vi "Text control 2 v6.8.vi"() -> ()   [LabVIEW 2016]
panel:
  in  "Tab Control":enum32{"Main", "Other parameters"}(tab)
  in  "Plot sample extrema vs time":bool
  out "Line running":i32
  out "Total lines":i32
  out "Path":path=path "C:/users/rlp38/09Apr2009LTtesting/test2.txt"
  out "I vs Vg":cluster{"Y data in":dbl[], "X data in":dbl[]}[](graph)
  out "Is max":dbl format="%.2e"
  out "Id max":dbl format="%.2e"
  out "Ig max":dbl format="%.2e"
  out "Imax vs time":cluster{"Y data in":dbl[], "X data in":dbl[]}[](graph)
  out "Imin vs time":cluster{"Y data in":dbl[], "X data in":dbl[]}[](graph)
  out "I vs Vd":cluster{"Y data in":dbl[], "X data in":dbl[]}[](graph)
  in  "Script":string="#pulsedstressV d 0.03 20 0 0.5 0.0827 5\n#\n#itime m\n#gaterangemode a\n#drainrangemode a\n#pulsed on 0.05 0 0.02\n#transfer d -10 40 1 5 40 35\n#transfer d -10 40 1 5 40 35\n#transfer d -10 40 1 5 40 35\n#output d 0 40 20 0 40 1\n#\n#\n#sample 1 0.008 221 6 0.003\n#samplei 400e-6 200 6 0.002 0.1\n#vsu2pulse -10 4\n#\n#stressV 0.016 0.03 2e-4 0.1e-3 11\n#stressI 220e-7 0.08 15\n#transfer s -1 1 0.5 -0.005 0.005 0.005\n#output s 0 0 0 -0.008 0.008 0.002"
  out "Command running:":string
  out "Serial port data":string
  out "Elapsed Time":dbl caption="Elapsed Time (s)"
  in  "Time Units":u16(ring)=1 items=["Seconds", "Minutes", "Hours"]
  in  "Time Offset":dbl caption="Set Start Time (s)"
  in  "Reset":bool
  in  "Auto Reset":bool
  in  "integration time":u32(slide) max=2 step=1 scale=0.0..2.0
  out "Is on":dbl format="%.2e"
  out "Id on":dbl format="%.2e"
  out "Ig on":dbl format="%.2e"
  out "Ion vs time":cluster{"Y data in":dbl[], "X data in":dbl[]}[](graph)
  out "Ioff vs time":cluster{"Y data in":dbl[], "X data in":dbl[]}[](graph)
  out "Ig min":dbl format="%.2e"
  out "Id min":dbl format="%.2e"
  out "Is min":dbl format="%.2e"
  out "Is off":dbl format="%.2e"
  out "Id off":dbl format="%.2e"
  out "Ig off":dbl format="%.2e"
  in  "Integration time (long)":dbl=0.32 min=0.04 max=2.0 step=0.02 format="%.2f"
  in  "Integration time (short)":dbl=0.0019 min=8e-05 max=0.0019 step=8e-05 format="%^.0e"
  in  "Drain: Compliance":dbl=0.001 format="%.8f"
  in  "Gate: Compliance":dbl=0.001 format="%.8f"
  in  "Interrupt scan":bool
  in  "Interrupt program":bool
  in  "Plot output curve extrema vs time":bool
  in  "Plot transfer curve extrema vs time":bool
  out "I vs time (Bias Stress)":cluster{"Y data in":dbl[], "X data in":dbl[]}[](graph)
  in  "Sample I - Probe 4 (Disabled)":u32(ring)=3 items=["SMU1  ", "SMU2  ", "SMU3  ", "SMU4  ", "SMU5  ", "SMU6  "]
  in  "Sample I - Source/Common":u32(ring) items=["SMU1  ", "SMU2  ", "SMU3  ", "SMU4  ", "SMU5  ", "SMU6  "]
  in  "Sample I - Probe 3 (Disabled)":u32(ring)=2 items=["SMU1  ", "SMU2  ", "SMU3  ", "SMU4  ", "SMU5  ", "SMU6  "]
  in  "Sample I - Drain/Gate":u32(ring)=1 items=["SMU1  ", "SMU2  ", "SMU3  ", "SMU4  ", "SMU5  ", "SMU6  "]
  in  "Sample - Probe 4":u32(ring)=3 items=["SMU1  ", "SMU2  ", "SMU3  ", "SMU4  ", "SMU5  ", "SMU6  "]
  in  "Sample - Source/Common":u32(ring) items=["SMU1  ", "SMU2  ", "SMU3  ", "SMU4  ", "SMU5  ", "SMU6  "]
  in  "Sample - Gate":u32(ring)=2 items=["SMU1  ", "SMU2  ", "SMU3  ", "SMU4  ", "SMU5  ", "SMU6  "]
  in  "Sample - Drain":u32(ring)=1 items=["SMU1  ", "SMU2  ", "SMU3  ", "SMU4  ", "SMU5  ", "SMU6  "]
  in  "Gate Range\nmode":u16(ring) items=["Auto", "Limited", "Fixed"]
  in  "Gate Range":u8(slide)=3 max=11 scale=0.0..11.0
  in  "Source/Drain\nRange mode":u16(ring) items=["Auto", "Limited", "Fixed"]
  in  "Source/Drain Range":u8(slide)=3 max=11 scale=0.0..11.0
  in  "Panel Controls":T1={"Emergency Stop"=refnum, "TransGraph Max"=1e-05, "Text/Graph (text=false)"=TRUE} {"TransGraph Max" format="%.2e"}
  in  "Panel Controls 2":T2={"Emergency Stop"=refnum, "TransGraph Max"=1e-05, "Text/Graph (text=false)"=TRUE, "TransGraph Min"=1e-11} {"TransGraph Min" format="%.2e"; "TransGraph Max" format="%.2e"}
  out "error out":errorcluster
  in  "Delay before read (ms)":u32=1000
  in  "byte count":u32=64
  in  "Serial End Mode for Reads":u16(ring)=2 items=["None", "LastBit", "TermChar"]
  in  "Timeout (ms)":u32=10000
  in  "Enable Termination\nChar (T)":bool=TRUE
  in  "Termination char\n(0xA = '\\n' = LF)\n(0xD = '\\r' = CR)":u8=13 format="%.0x"
  in  "flow control":u16(ring) items=["None"=0, "XON/XOFF"=1, "RTS/CTS"=2, "DTR/DSR"=4]
  in  "stop bits":u16(ring)=10 items=["1.0"=10, "1.5"=15, "2.0"=20]
  in  "parity":u16(ring) items=["None", "Odd", "Even", "Mark", "Space"]
  in  "data bits":u16=8 min=5 max=8 step=1
  in  "VISA resource name":refnum<visa-resource-name>="COM6"
  in  "baud rate":u32=9600
  out "Timings Indicator":T3
  in  "Timings (overwritten by the Front Panel)":T4={"integration time"=0, "Short/Long integration time"=0.00064, "hold time (sec)"=0.0, "delay time (sec)"=0.0, "Step Time (0 disables)"=0.0, "sweep method"=0, "Pulse period"=0.005, "Base voltage"=0.0, "Pulse width"=0.0005} {"Pulse width" min=0.0005 max=0.1 step=0.0001 format="%.4f"; "Base voltage" format="%^.4e"; "Pulse period" min=0.005 max=1.0 step=0.0001 format="%.4f"; "sweep method" items=["Continuous", "Pulsed"]; "Step Time (0 disables)" format="%.2f"; "delay time (sec)" format="%.4f"; "hold time (sec)" format="%.4f"; "Short/Long integration time" format="%^.0e"; "integration time" scale=0.0..2.0}
  in  "Probe 4":cluster{"on/off":bool, "Voltage":dbl} {"Voltage" min=-100.0 max=100.0 format="%.2f"}
  in  "Full Reset":bool
  in  "Standby":T5
  out "Probe 4 Indicator":cluster{"on/off":bool, "Voltage":dbl} {"Voltage" min=-100.0 max=100.0 format="%.2f"}
  in  "Transfer/Output - Drain":u32(ring)=1 items=["SMU1  ", "SMU2  ", "SMU3  ", "SMU4  ", "SMU5  ", "SMU6  "]
  in  "Transfer/Output - Gate":u32(ring)=2 items=["SMU1  ", "SMU2  ", "SMU3  ", "SMU4  ", "SMU5  ", "SMU6  "]
  in  "Transfer/Output - Source/Common":u32(ring) items=["SMU1  ", "SMU2  ", "SMU3  ", "SMU4  ", "SMU5  ", "SMU6  "]
  in  "Transfer/Output - Probe 4":u32(ring)=3 items=["SMU1  ", "SMU2  ", "SMU3  ", "SMU4  ", "SMU5  ", "SMU6  "]
  in  "Pulsed Stress V - Probe 4":u32(ring)=3 items=["SMU1  ", "SMU2  ", "SMU3  ", "SMU4  ", "SMU5  ", "SMU6  "]
  in  "Pulsed Stress V - Vextra":u32(ring)=1 items=["VSU1  ", "VSU2  "]
  in  "Pulsed Stress V - Drain":u32(ring)=1 items=["SMU1  ", "SMU2  ", "SMU3  ", "SMU4  ", "SMU5  ", "SMU6  "]
  in  "Pulsed Stress V - Source/Common":u32(ring) items=["SMU1  ", "SMU2  ", "SMU3  ", "SMU4  ", "SMU5  ", "SMU6  "]
  in  "Pulsed Stress V - Gate":u32(ring)=2 items=["SMU1  ", "SMU2  ", "SMU3  ", "SMU4  ", "SMU5  ", "SMU6  "]
  in  "FPP - Drain":u32(ring)=1 items=["SMU1  ", "SMU2  ", "SMU3  ", "SMU4  ", "SMU5  ", "SMU6  "]
  in  "FPP - Gate":u32(ring)=2 items=["SMU1  ", "SMU2  ", "SMU3  ", "SMU4  ", "SMU5  ", "SMU6  "]
  in  "FPP - Probe 1":u32(ring) items=["SMU1  ", "SMU2  ", "SMU3  ", "SMU4  ", "SMU5  ", "SMU6  "]
  in  "FPP - Probe 2":u32(ring)=3 items=["SMU1  ", "SMU2  ", "SMU3  ", "SMU4  ", "SMU5  ", "SMU6  "]
  in  "FPP - Source":u32(ring) items=["VSU1  ", "VSU2  "]
  in  "Stress V - Drain":u32(ring)=1 items=["SMU1  ", "SMU2  ", "SMU3  ", "SMU4  ", "SMU5  ", "SMU6  "]
  in  "Stress V - Gate":u32(ring)=2 items=["SMU1  ", "SMU2  ", "SMU3  ", "SMU4  ", "SMU5  ", "SMU6  "]
  in  "Stress V - Source/Common":u32(ring) items=["SMU1  ", "SMU2  ", "SMU3  ", "SMU4  ", "SMU5  ", "SMU6  "]
  in  "Stress I - Drain/Gate":u32(ring)=1 items=["SMU1  ", "SMU2  ", "SMU3  ", "SMU4  ", "SMU5  ", "SMU6  "]
  in  "Stress I - Source/Common":u32(ring) items=["SMU1  ", "SMU2  ", "SMU3  ", "SMU4  ", "SMU5  ", "SMU6  "]
  in  "VSU2 Stress - Source/Common":u32(ring) items=["SMU1  ", "SMU2  ", "SMU3  ", "SMU4  ", "SMU5  ", "SMU6  "]
  in  "VISA resource name in":refnum<visa-resource-name>="GPIB0::14::INSTR"
  in  "Gate":T6={"Gate Start"=0.0, "Gate Stop"=2.0, "Gate Step (linear only)"=1.0, "Gate Compliance"=0.0001, "Gate PComp"=0.0, "Range mode"=0, "Range"=6} {"Range" max=11 scale=0.0..11.0; "Range mode" items=["Auto", "Limited", "Fixed"]; "Gate PComp" format="%^.2e"; "Gate Compliance" format="%^.2e"; "Gate Step (linear only)" format="%^.4e"; "Gate Stop" format="%^.4e"; "Gate Start" format="%^.4e"}
  in  "Drain 2":T7={"Drain Start"=0.0, "Drain Stop"=2.0, "Drain Compliance"=0.0001, "Drain Step"=1.0, "Drain PComp"=0.0, "Range mode"=0, "Range"=6} {"Range" max=11 scale=0.0..11.0; "Range mode" items=["Auto", "Limited", "Fixed"]; "Drain PComp" format="%^.2e"; "Drain Step" format="%^.4e"; "Drain Compliance" format="%^.2e"; "Drain Stop" format="%^.4e"; "Drain Start" format="%^.4e"}
  # "Time"
  # "Syntax:\nitime [s|m|l] time(sec): [s|m|l] determines the integration time setting (small|medium|long) and time sets the value.\nNOTE: The value of the integration time has to be within the range allowed by its category (s|m|l), otherwise, the closest value will be used. (e.g. if the category is set to short but the time value is very long, the actual value used will be the maximum short integration time.\nIntegration times:\n    Short: Default: 640 us. Range: 8E-5 - 1.92E-3 seconds.\n    Medium: Fixed at 1 NPL cycle (0.02 seconds).\n    Long: Default: 16 NPL cycles (0.32 seconds). Range: 2-100 NPL cycles (0.04 seconds - 2 seconds).\ngaterangemode [a|l|f]\ndrainrangemode [a|l|f]\npulsed [on|off] PulsePeriod(sec) PulseBaseVoltage PulseONWidth(sec)\nstandby [on l off]\nwait NumMilliseconds\nwait-min NumMinutes\n# texthere = comment\nProbe4 [ON|OFF] Voltage\ntransfer [s|d] VgStart VgStop VgStep VdStart VdStop VdStep\noutput [s|d] VgStart VgStop VgStep VdStart VdStop VdStep\nsample Vg Vd NumSamples Time(s) SampleInterval(s)\nsamplei Idg NumSamples Time(s) SampleInterval(s) VDGcompliance\n100 samples is approximately 13 seconds with medium integration\n# if in doubt use SampleInterval(s) = 0.004\n    NOTE: When doing bias stress measurements, set the Time Units to \"Seconds\", as the \"sample\" command has been configured to give the output to seconds.\nstressV VG VD IGcompliance IDcompliance Duration(sec)\nstressI IDG VDGcompliance Duration(sec)\nvsu2pulse Bias Duration(s)\npulsedstressV [s|d] VEstop VgON VgOFF Period(s) PulseONwidth(s) Vd\nsample-fpp Vg Vd NumSamples Time\nresample-fpp Vg Vd\ntransfer-fpp [s|d] VgStart VgStop VgStep VdStart VdStop VdStep\noutput-fpp [s|d] VgStart VgStop VgStep VdStart VdStop VdStep\nserial SerialPortCommand"
  # "1\n2\n3\n4\n5\n6\n7\n8\n9\n10\n11\n12\n13\n14\n15\n16\n17\n18\n19\n20"
  # "SMUs"
  # "Serial port settings"
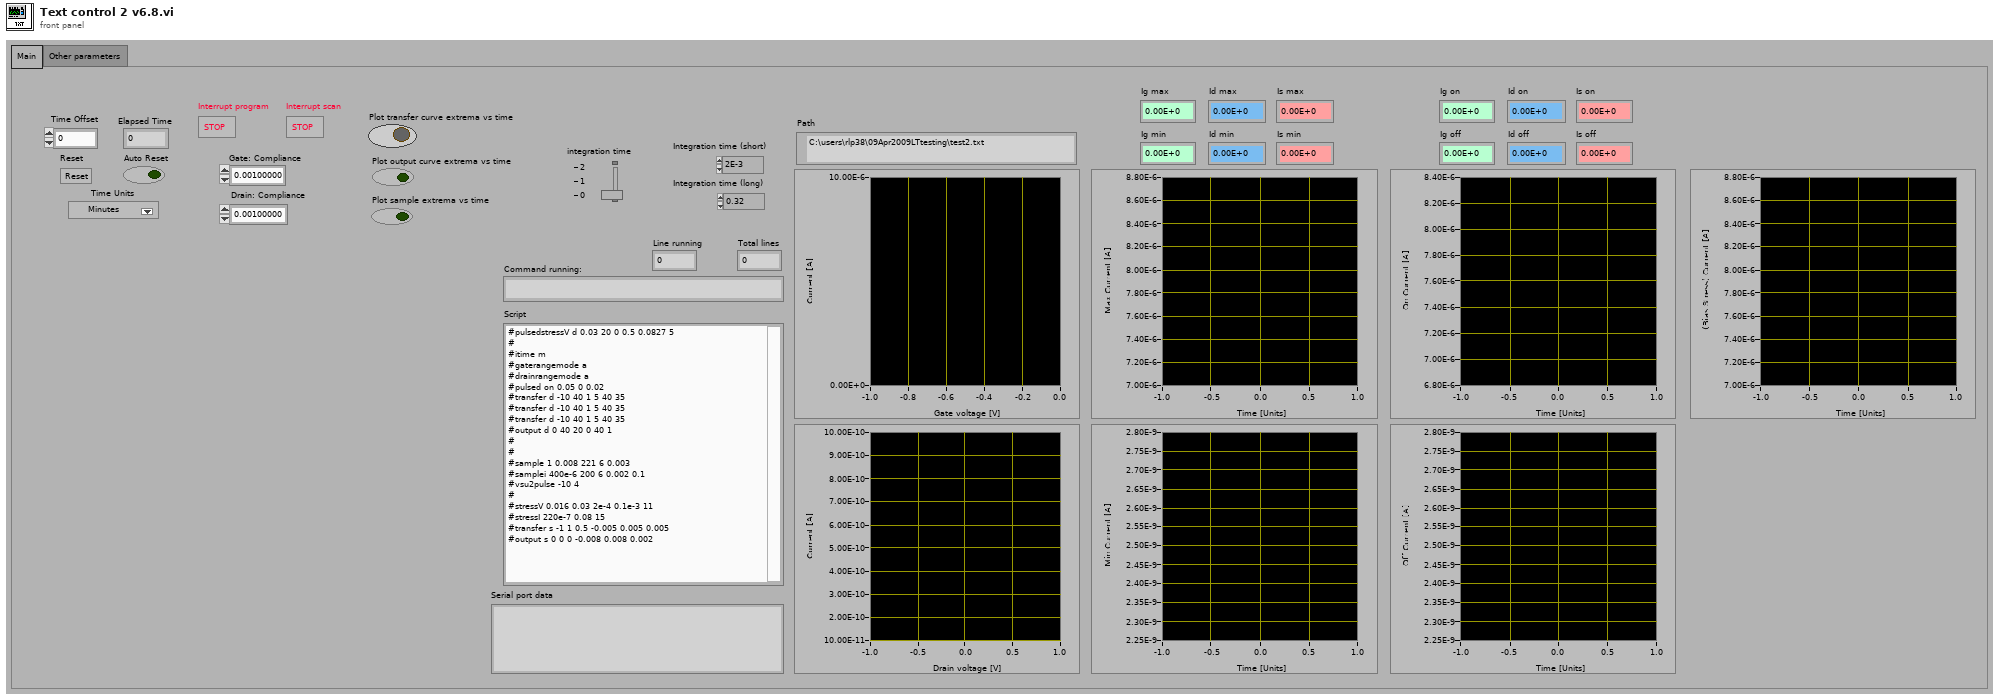
[diagram p1: front panel]
types:
  T1 = cluster{"Emergency Stop":refnum<vi>, "TransGraph Max":dbl, "Text/Graph (text=false)":bool}
  T2 = cluster{"Emergency Stop":refnum<vi>, "TransGraph Max":dbl, "Text/Graph (text=false)":bool, "TransGraph Min":dbl}
  T3 = cluster{"integration time (0:s, 1:m, 2:l)":u32, "Short/Long integration time":dbl, "hold time (sec)":dbl, "delay time (sec)":dbl, "Step Time (0 disables)":dbl, "sweep method":u16, "Pulse period":dbl, "Base voltage":dbl, "Pulse width":dbl}
  T4 = cluster{"integration time":u32, "Short/Long integration time":dbl, "hold time (sec)":dbl, "delay time (sec)":dbl, "Step Time (0 disables)":dbl, "sweep method":u16, "Pulse period":dbl, "Base voltage":dbl, "Pulse width":dbl}
  T5 = cluster{"Gate Standby":bool, "Drain Standby":bool}
  T6 = cluster{"Gate Start":dbl, "Gate Stop":dbl, "Gate Step (linear only)":dbl, "Gate Compliance":dbl, "Gate PComp":dbl, "Range mode":u16, "Range":u8}
  T7 = cluster{"Drain Start":dbl, "Drain Stop":dbl, "Drain Compliance":dbl, "Drain Step":dbl, "Drain PComp":dbl, "Range mode":u16, "Range":u8}
  T8 = enum16{"open", "replace", "create", "open or create", "replace or create", "replace or create with confirmation"}
  T9 = cluster{"V2 Start":dbl, "V2 Step":dbl, "Number of points":i32}
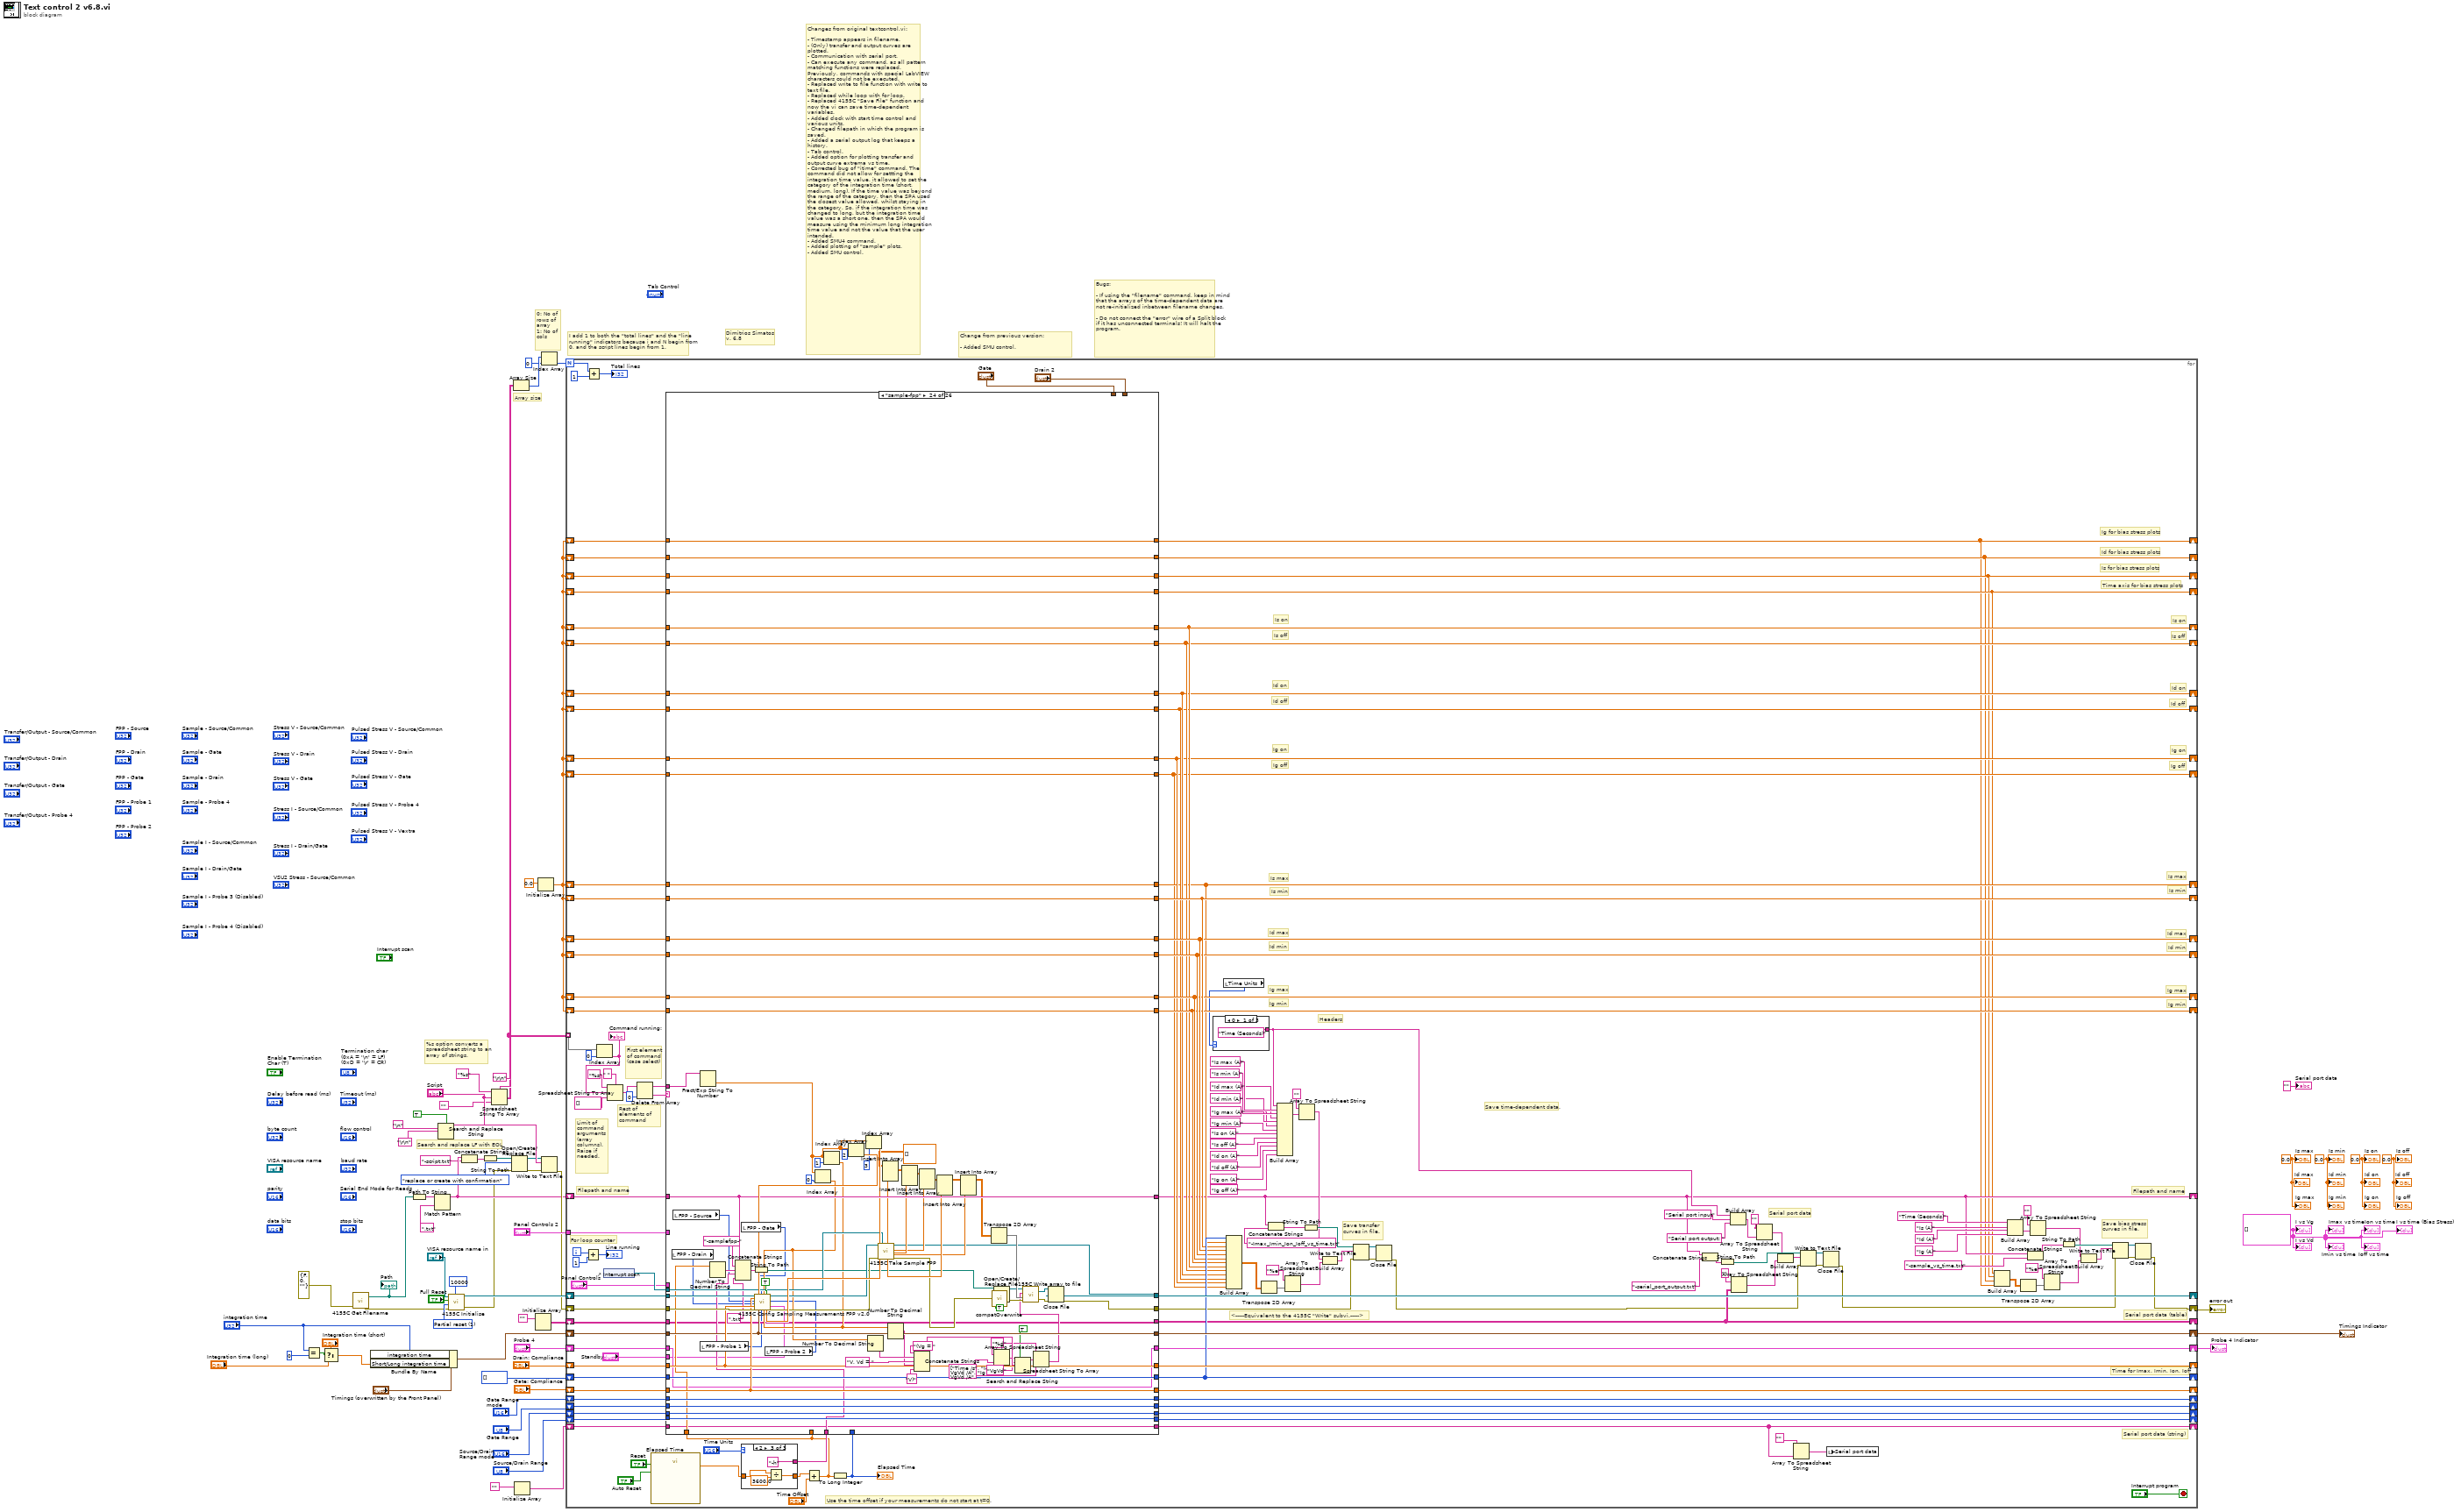
[diagram p0: block diagram]
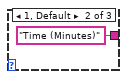
[diagram p2: hidden frame]
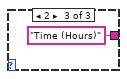
[diagram p3: hidden frame]
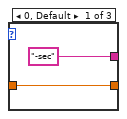
[diagram p4: hidden frame]
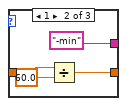
[diagram p5: hidden frame]
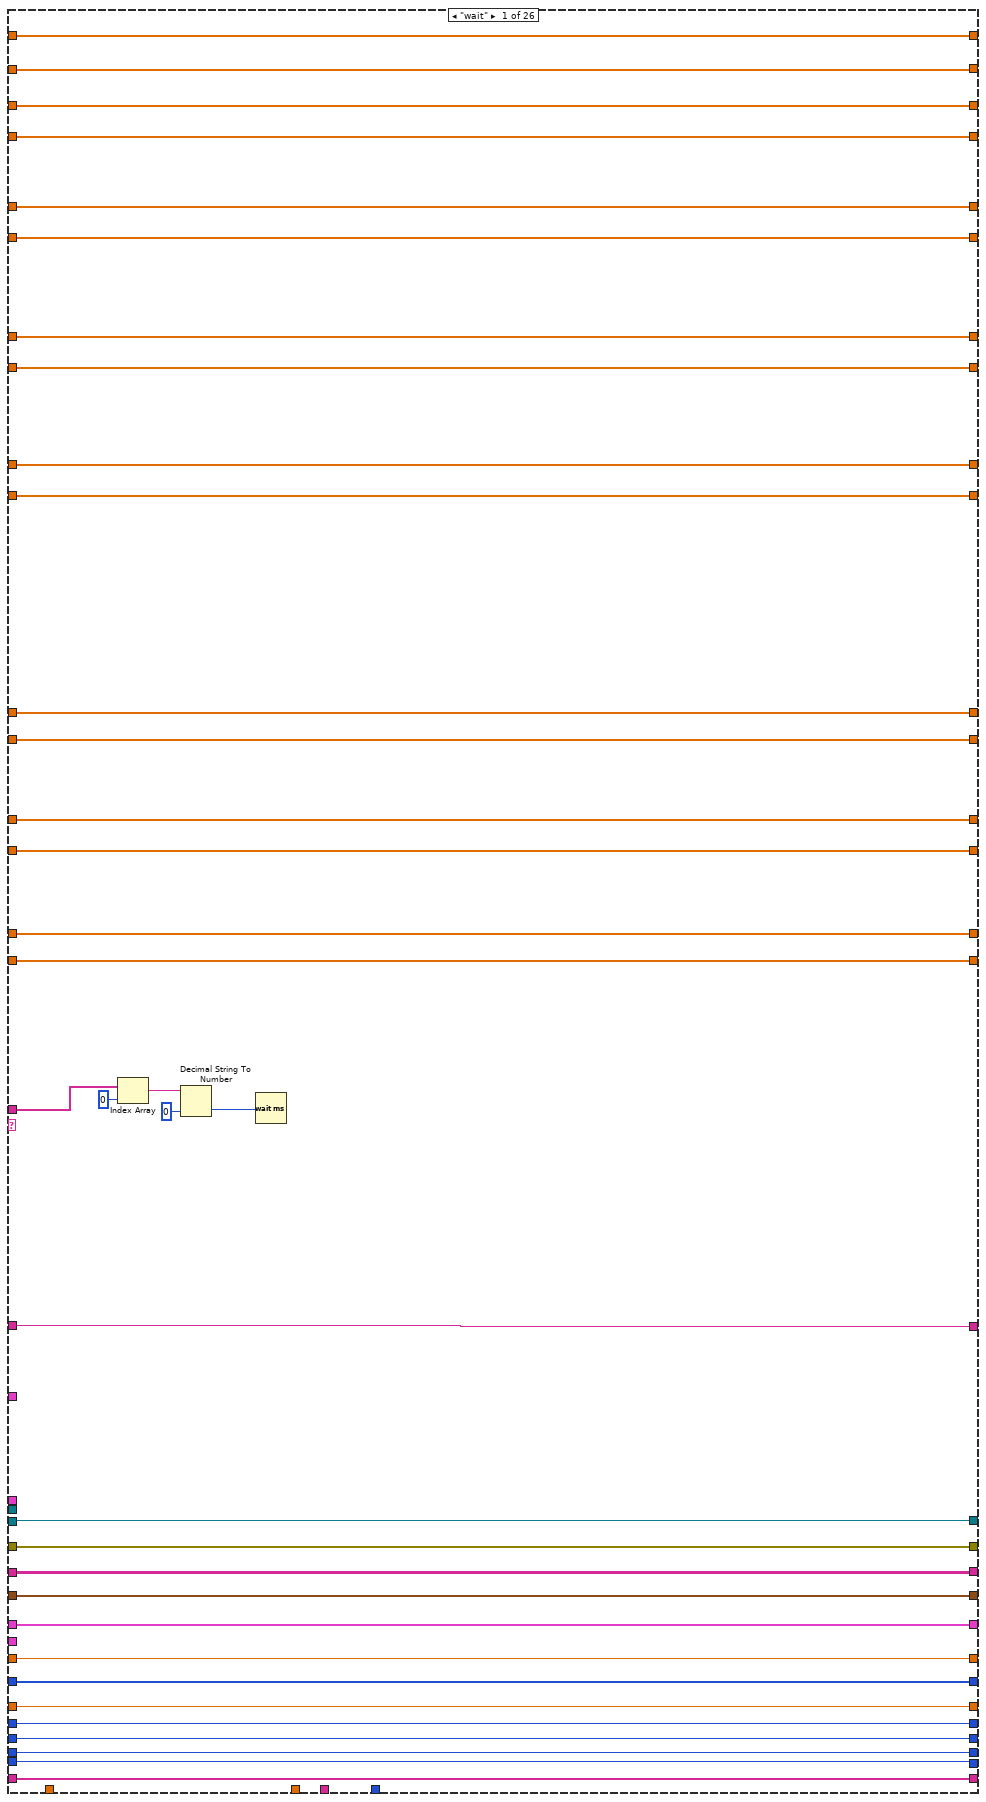
[diagram p6: hidden frame]
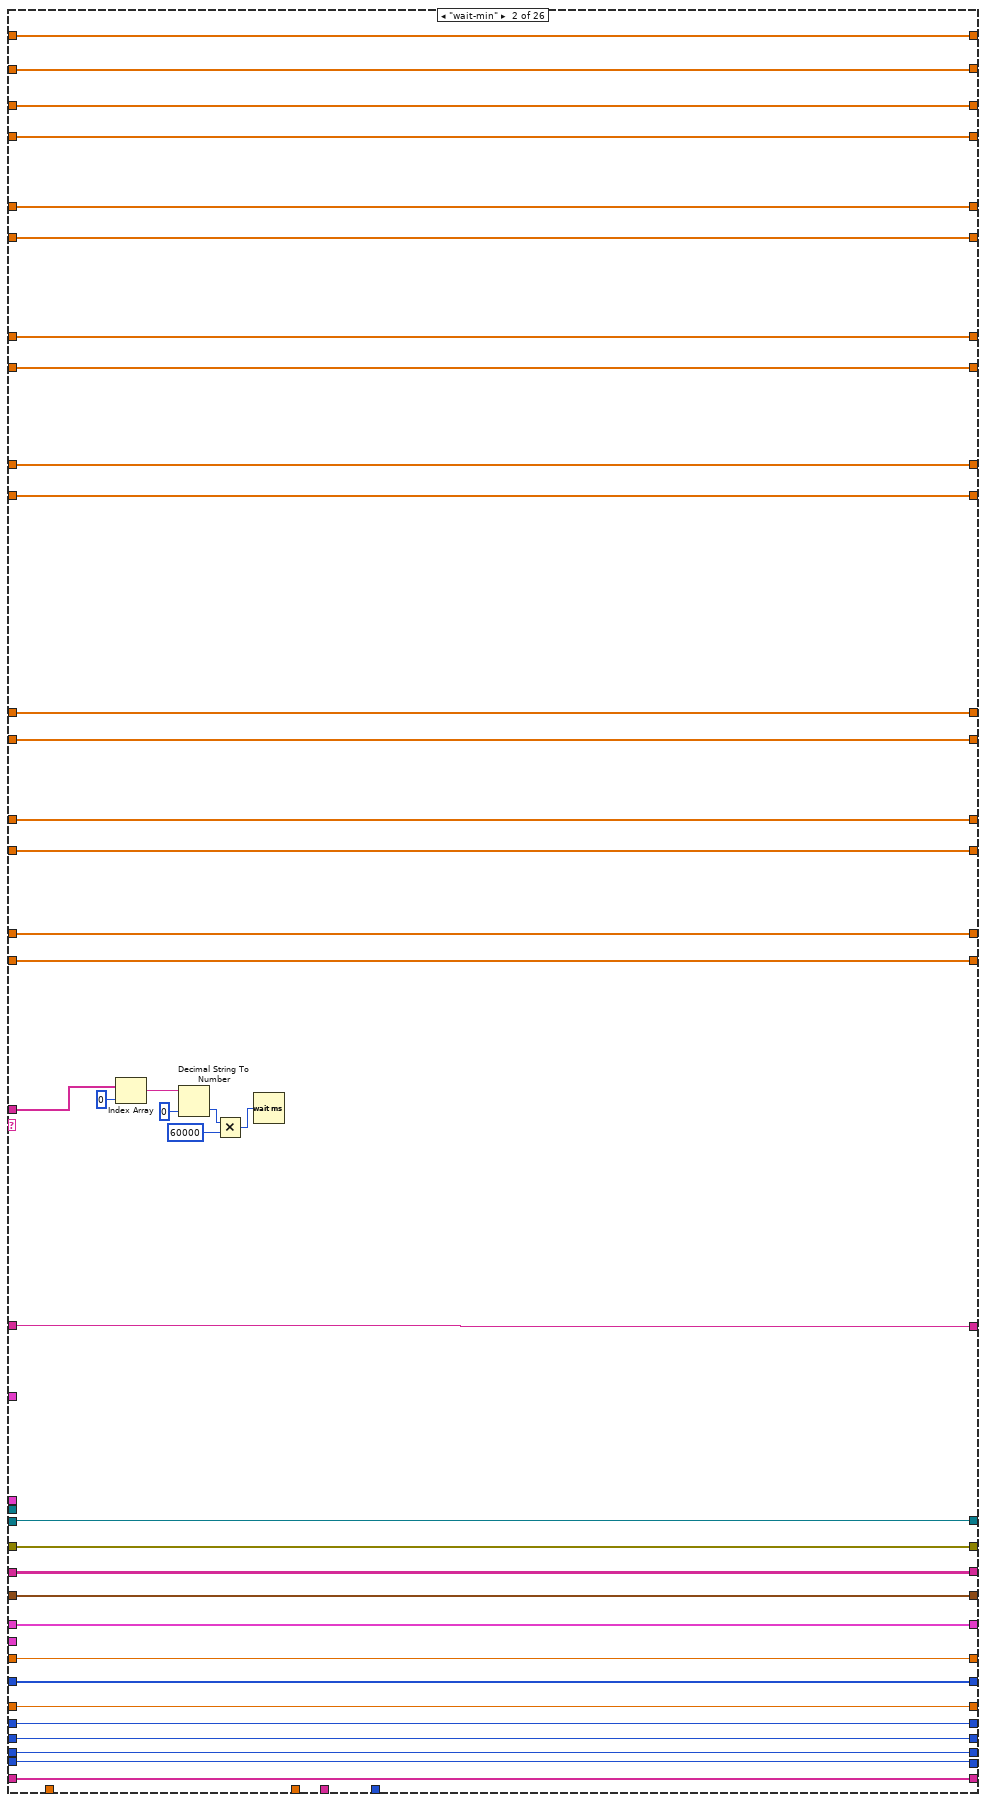
[diagram p7: hidden frame]
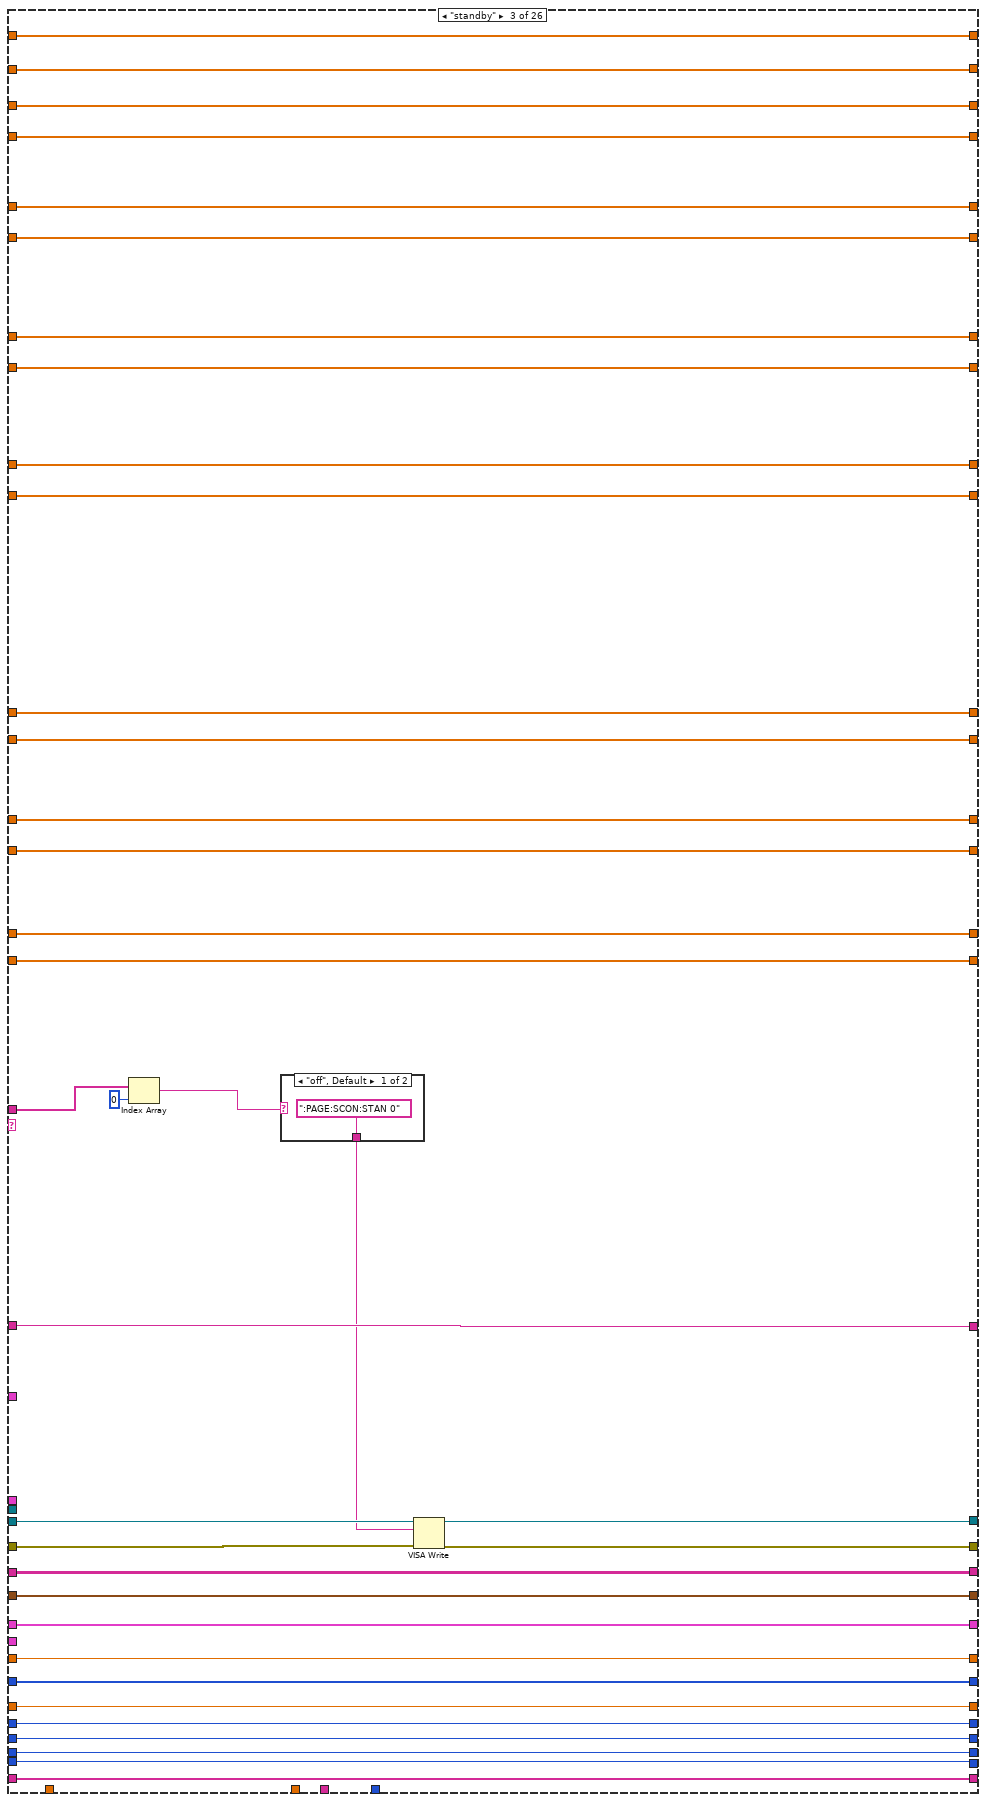
[diagram p8: hidden frame]
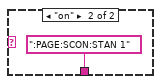
[diagram p9: hidden frame]
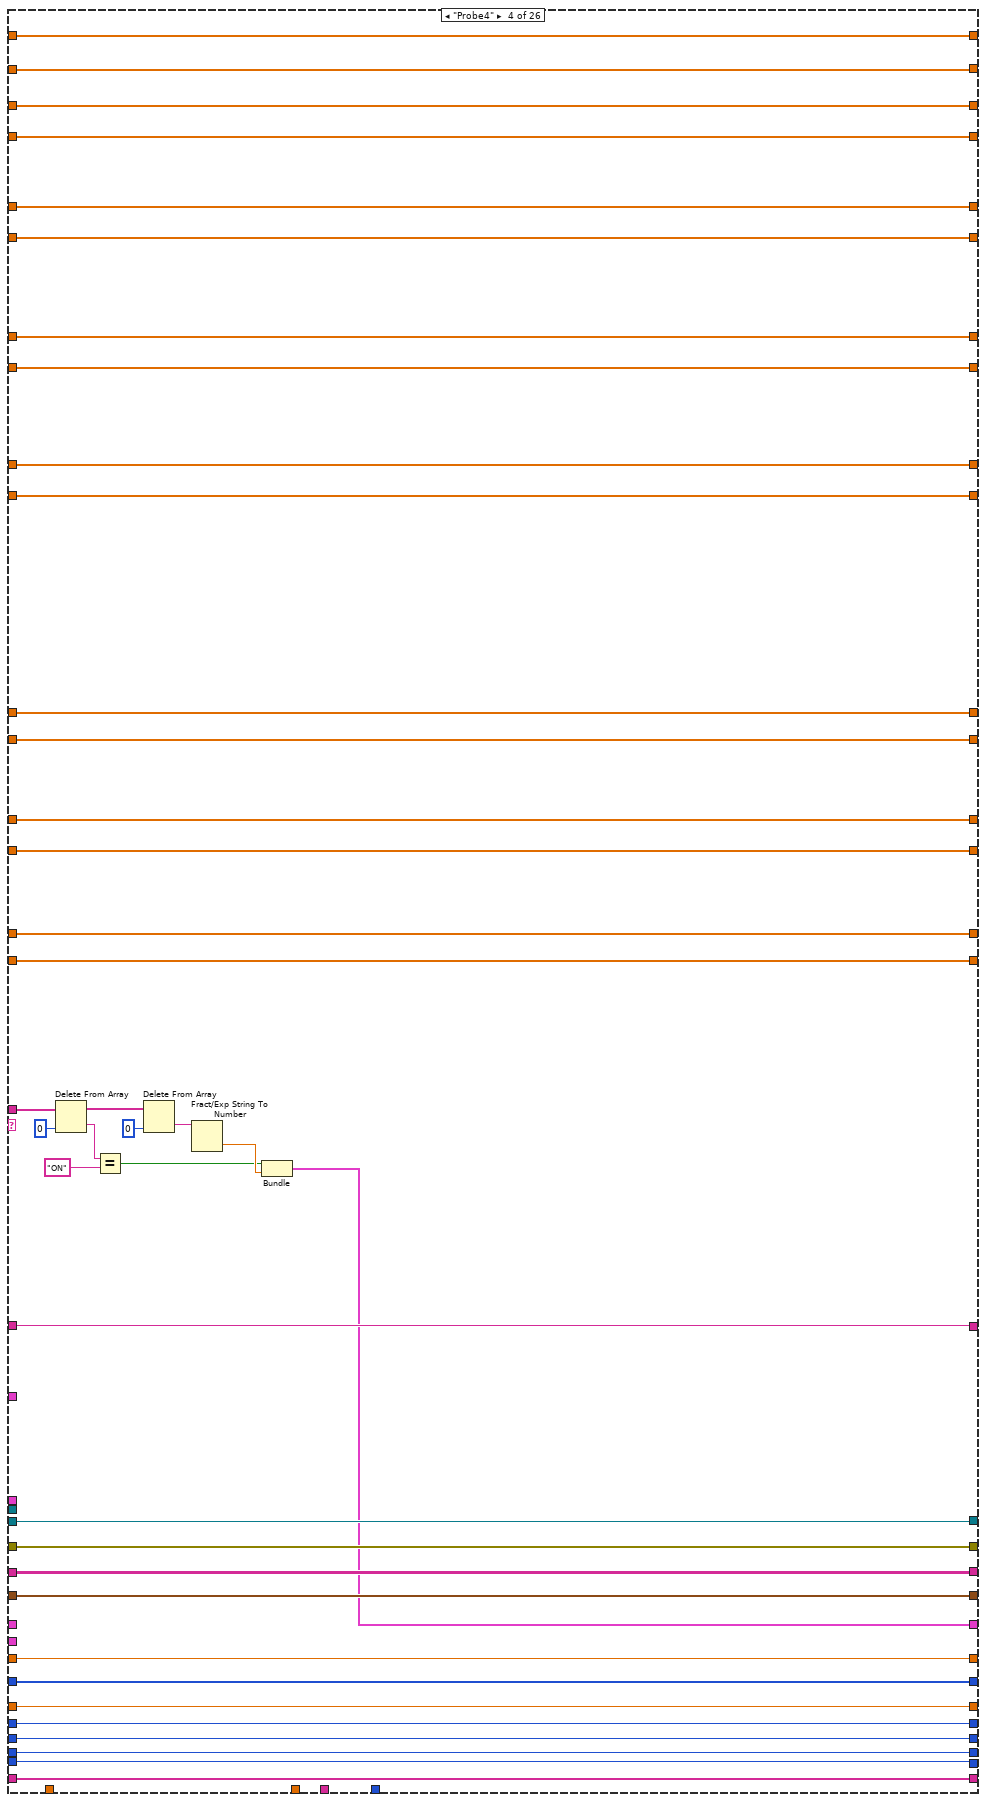
[diagram p10: hidden frame]
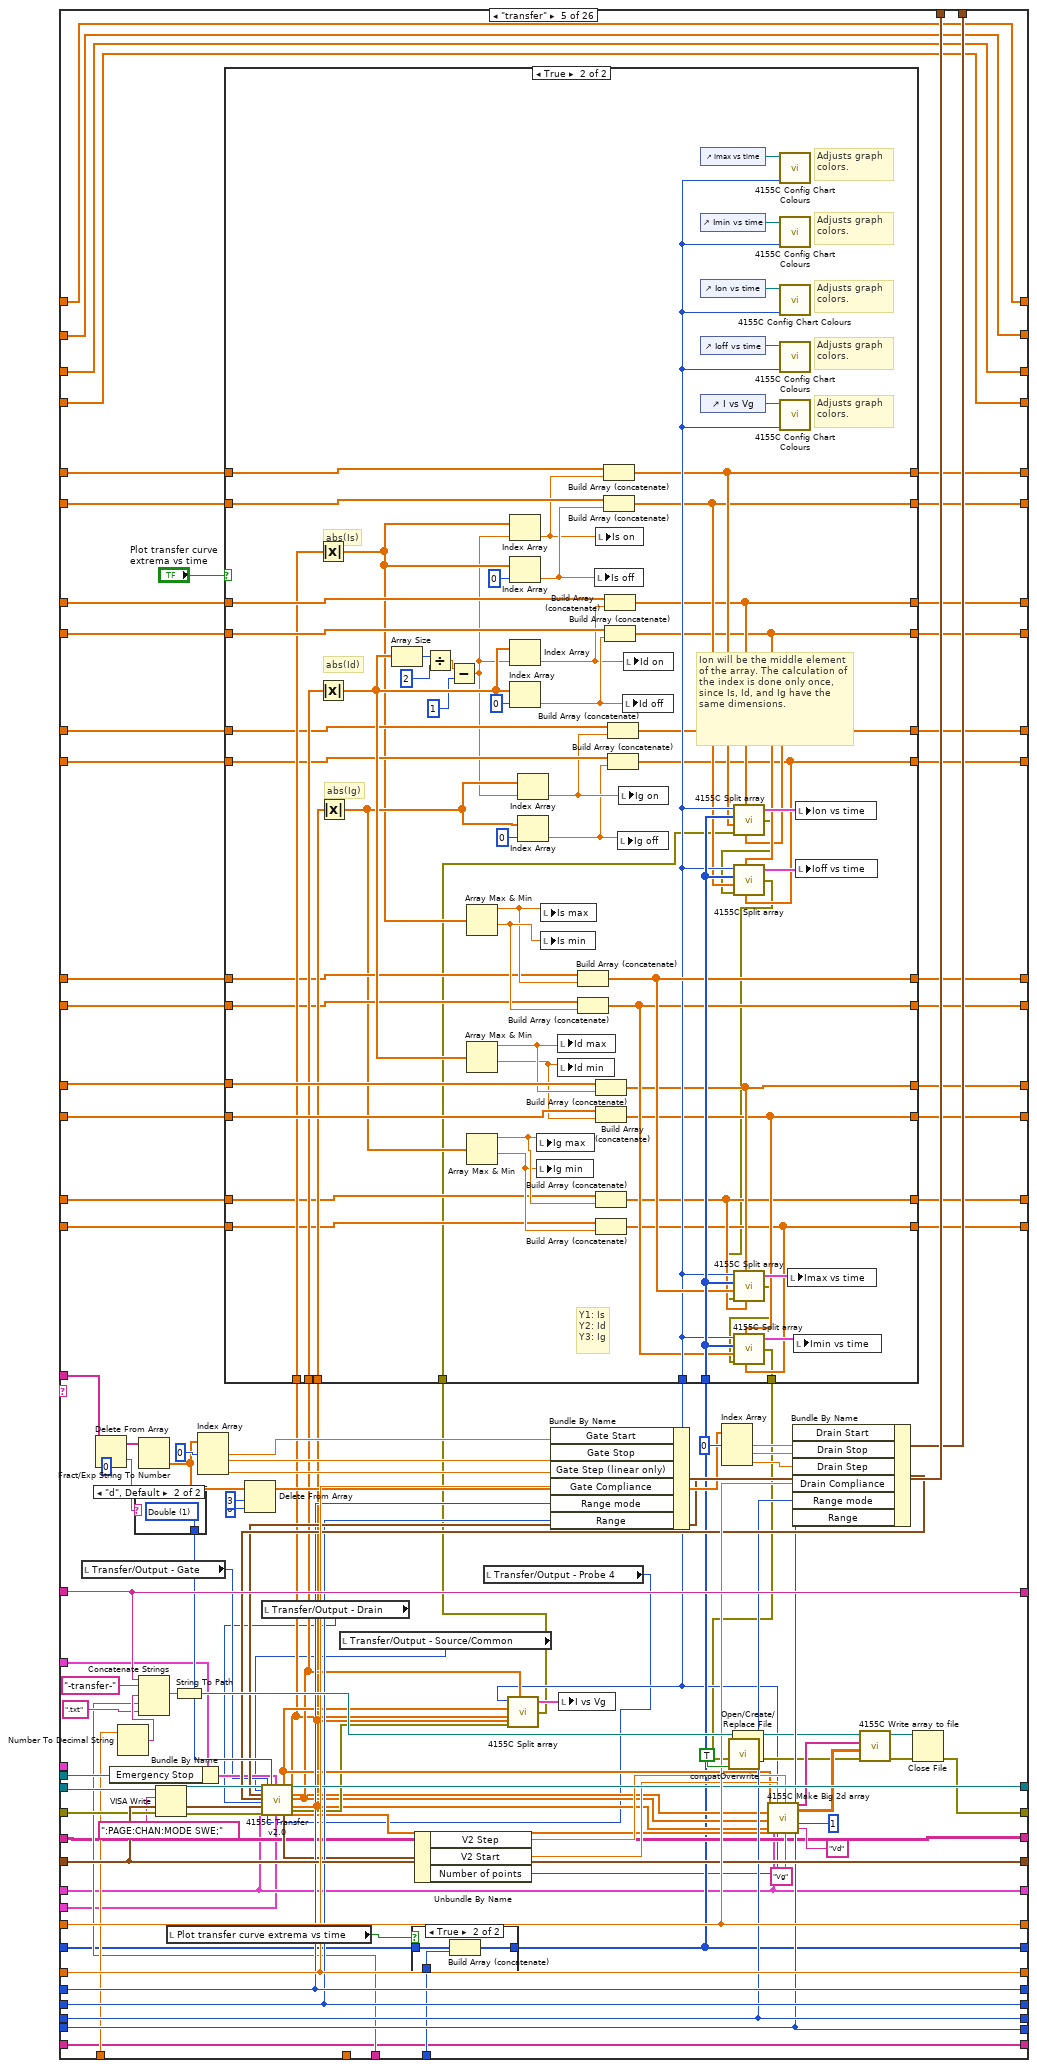
[diagram p11: hidden frame]
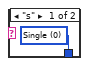
[diagram p14: hidden frame]
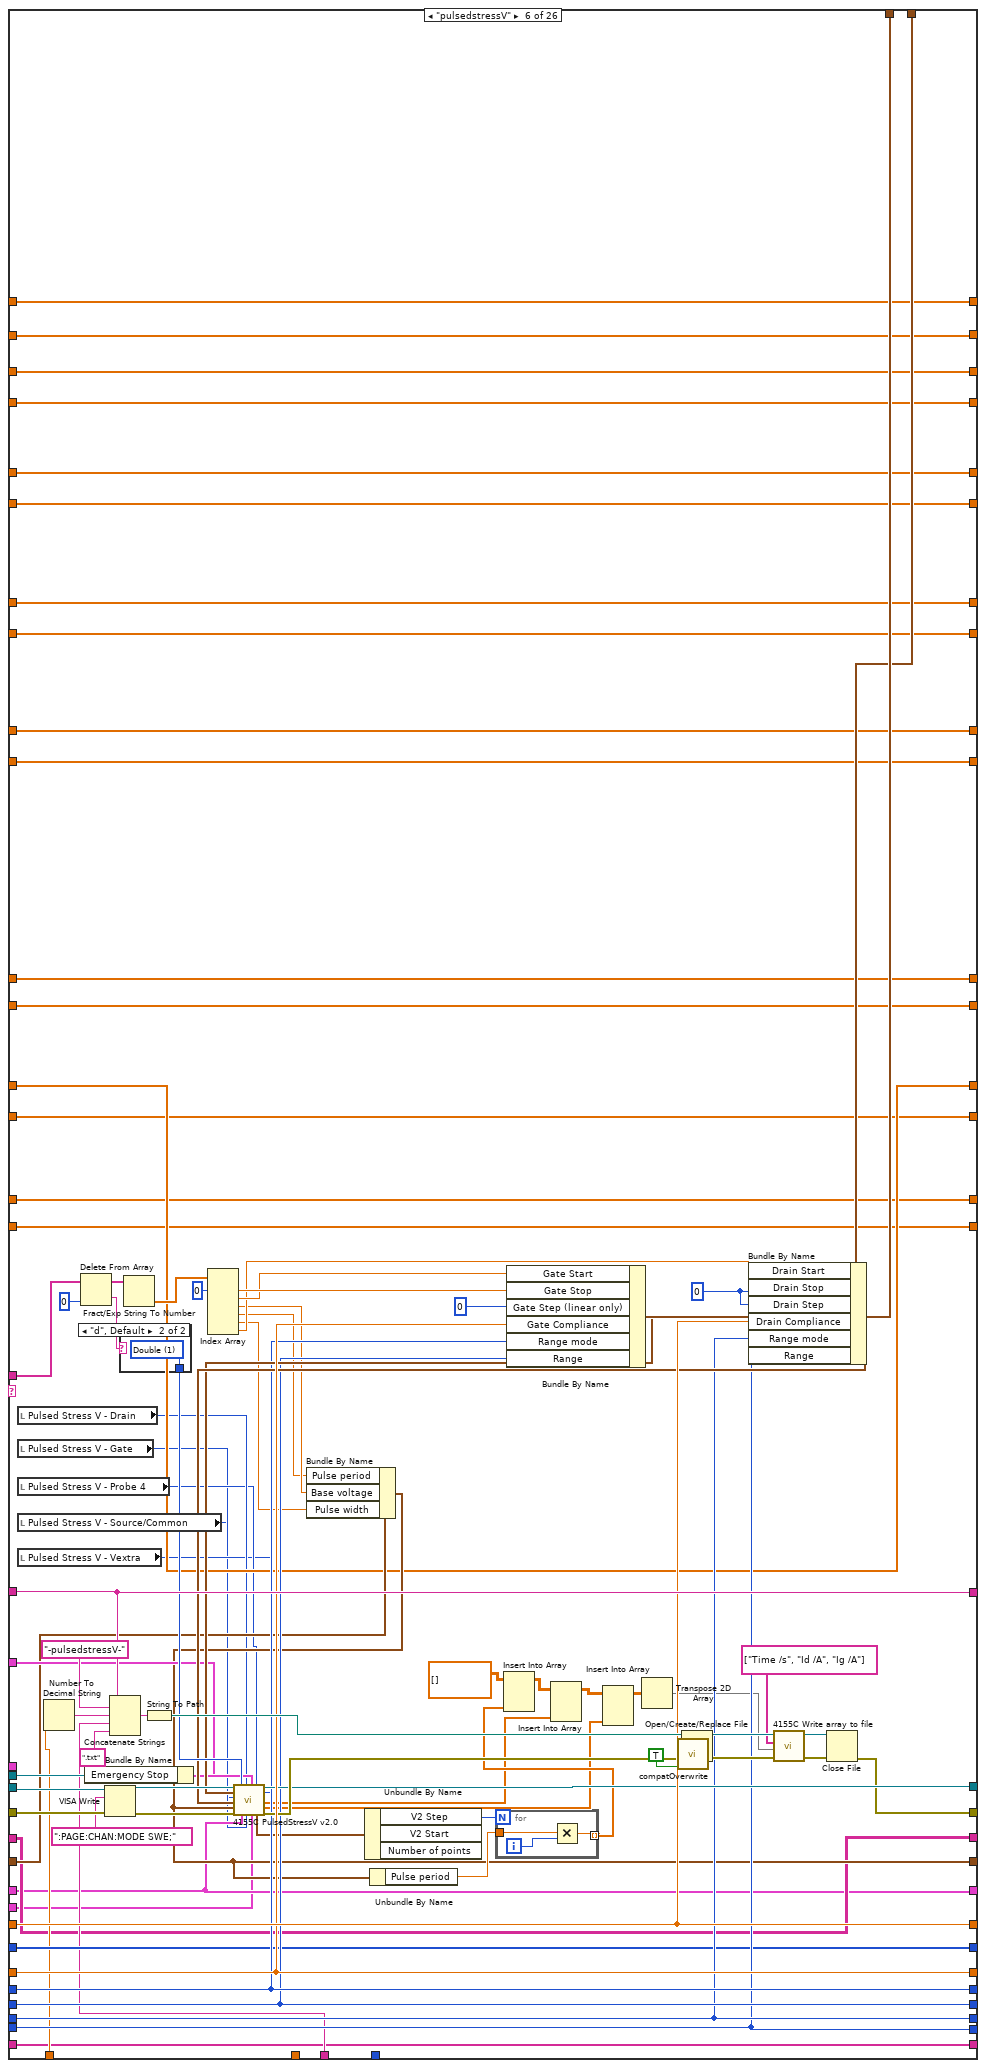
[diagram p15: hidden frame]
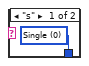
[diagram p16: hidden frame]
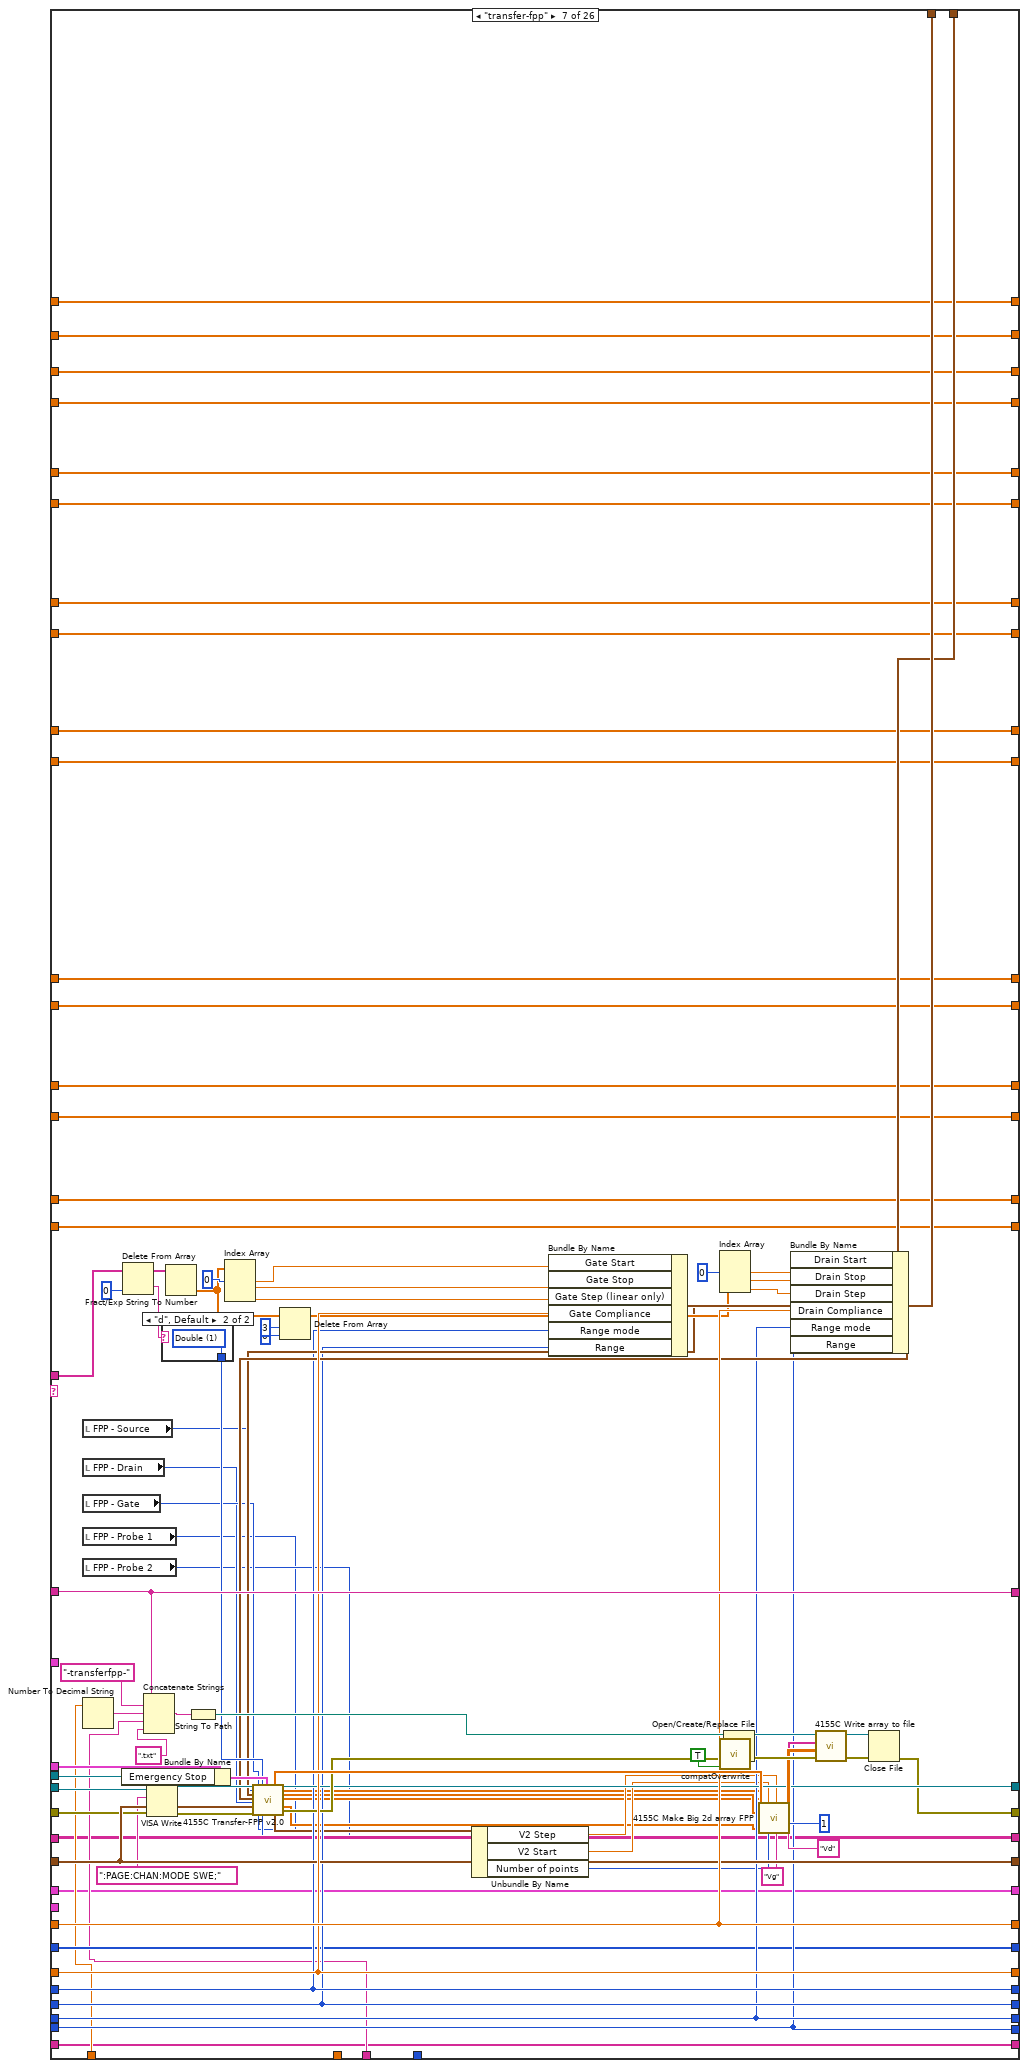
[diagram p17: hidden frame]
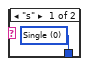
[diagram p18: hidden frame]
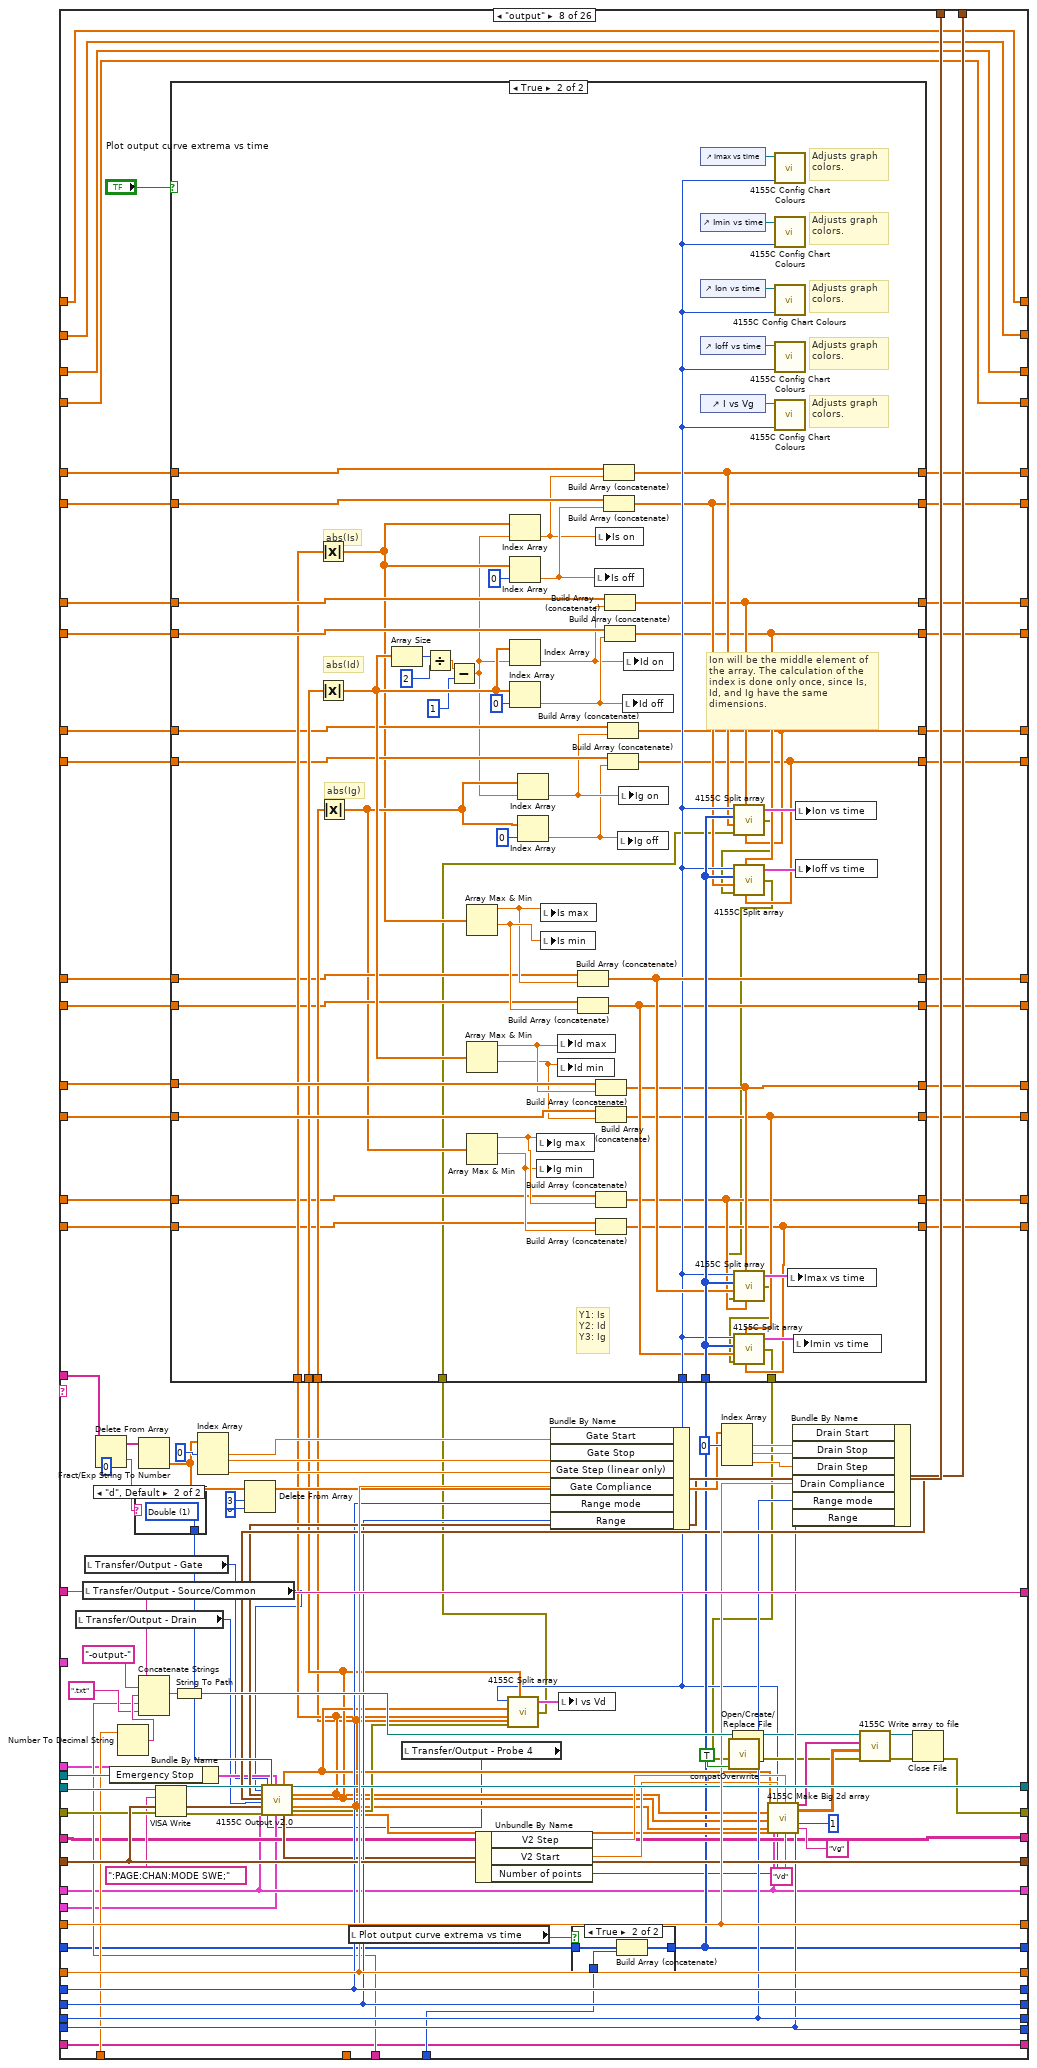
[diagram p19: hidden frame]
diagram:
  w2 = cluster{"Y data in":dbl[], "X data in":dbl[]}[] [] ("I vs Vg")
  w10 = 0.0 ("Is off")
  w11 = 0.0 ("Is on")
  w12 = 0.0 ("Is min")
  w13 = 0.0 ("Is max")
  w58 = u16 1 items=["Reset All", "Partial reset"] ("Type of reset")
  # "Change from previous version:\n\n- Added SMU control."
  # "I add 1 to both the \"total lines\" and the \"line running\" indicators because i and N begin from 0, and the script lines begin from 1."
  # "Bugs:\n\n- If using the \"filename\" command, keep in mind that the arrays of the time-dependent data are not re-initialized inbetween filename changes. \n\n- Do not connect the \"error\" wire of a Split block if it has unconnected terminals! It will halt the program."
  # "Array size"
  # "%s option converts a spreadsheet string to an array of strings."
  # "0: No of rows of array\n1: No of cols"
  # "Dimitrios Simatos\nv. 6.8"
  # "Changes from original textcontrol.vi:\n\n- Timestamp appears in filename.\n- (Only) transfer and output curves are plotted.\n- Communication with serial port.\n- Can execute any command, as all pattern matching functions were replaced. Previously, commands with special LabVIEW characters could not be executed.\n- Replaced write to file function with write to text file.\n- Replaced while loop with for loop.\n- Replaced 4155C \"Save File\" function and now the vi can save time-dependent variables.\n- Added clock with start time control and various units.\n- Changed filepath in which the program is saved.\n- Added a serial output log that keeps a history.\n- Tab control.\n- Added option for plotting transfer and output curve extrema vs time.\n- Corrected bug of \"itime\" command. The command did not allow for settting the integration time value, it allowed to set the category of the integration time (short, medium, long). If the time value was beyond the range of the category, then the SPA used the closest value allowed, whilst staying in the category. So, if the integration time was changed to long, but the integration time value was a short one, then the SPA would measure using the minimum long integration time value and not the value that the user intended.\n- Added SMU4 command.\n- Added plotting of \"sample\" plots.\n- Added SMU control."
  # "Search and replace LF with EOL"
  n1 = Equal?(x="integration time", y=u32 0) -> (x = y?=w59:bool)
  n2 = Select(t="Integration time (short)", s=w59, f="Integration time (long)") -> (s? t:f=w18:dbl)
  n3 = call "4155C Get Filename.vi"("error in (no error)"=errorcluster {"status"=FALSE, "code"=0, "source"=""}) -> ("error out"=w53:errorcluster, "path"=w28:path)  [unwired: 2 in, 1 out]
  "Path" <- w28
  n4 = Bundle By Name(cluster="Timings (overwritten by the Front Panel)", "integration time"="integration time", "Short/Long integration time"=w18) -> (w51:T4)
  n5 = Path To String(path=w28) -> (string=w29:string)
  n6 = Match Pattern(string=w29, regular expression=".txt") -> (before substring=w16:string)  [unwired: 1 in, 3 out]
  n7 = Search and Replace String(replace all?=TRUE ("replace all? (F)"), input string="Script", search string="\n", replace string="\r\n") -> (result string=w41:string)  [unwired: 4 in, 3 out]
  n8 = call "4155C Initialise.vi"("VISA resource name in"="VISA resource name in", "Reset"="Full Reset", "Type of reset"=w58, "error in (no error)"=w53, "VISA Timeout Value"=u32 10000) -> ("VISA Resource Name out"=w52:refnum<visa-resource-name>, "error out"=w8:errorcluster)
  n9 = Concatenate Strings(w16, "-script.txt" ("string")) -> (w17:string)
  n10 = String To Path(string=w17) -> (path=w6:path)
  n11 = Spreadsheet String To Array(delimiter (Tab)="\r\n", format string="%s", spreadsheet string="Script", array type (2D Dbl)="") -> (array=w32:string[][])
  n12 = Open/Create/Replace File(file path (use dialog)=w6, error in=w8, operation (0:open)=T8."replace or create with confirmation") -> (refnum out=w5:refnum<file>, error out=w7:errorcluster)  [unwired: 3 in, 1 out]
  n13 = Array Size(array=w32) -> (size(s)=w36:i32[])
  n14 = Initialize Array("") -> (w22:string[])  [unwired: 1 in]
  n15 = Initialize Array("") -> (w20:string[][])  [unwired: 2 in]
  n16 = Initialize Array(0.0 ("element")) -> (w1:dbl[])  [unwired: 1 in]
  n17 = Index Array(array=w36, index=0) -> (element=w34:i32)
  n18 = Write to Text File(file (use dialog)=w5, text=w41, error in=w7) -> (error out=w25:errorcluster)  [unwired: 1 in, 2 out]
  n19 = for {
    N: w34 -> [w160]
    shift-left: "Source/Drain Range" -> [w200]
    shift-right: [w196] -> _
    shift-left: "Source/Drain\nRange mode" -> [w201]
    shift-right: [w197] -> _
    shift-left: "Gate Range" -> [w202]
    shift-right: [w198] -> _
    shift-left: "Gate Range\nmode" -> [w203]
    shift-right: [w199] -> _
    shift-left: "Gate: Compliance" -> [w212]
    shift-right: [w208] -> _
    shift-left: "Drain: Compliance" -> [w213]
    shift-right: [w209] -> _
    shift-left: w51 -> [w214]
    shift-right: [w210] -> w19
    shift-left: w25 -> [w215]
    shift-right: [w70] -> w27
    shift-left: w52 -> [w216]
    shift-right: [w211] -> _
    shift-left: w16 -> [w217]
    shift-right: [w69] -> _
    tunnel: "Panel Controls 2" -> [w194]
    shift-right: [w112] -> _
    shift-left: w1 -> [w193]
    shift-right: [w147] -> _
    shift-left: i32[] [] -> [w189]
    tunnel: w32 -> [w188] mode=indexing
    shift-right: [w111] -> _
    shift-left: w1 -> [w165]
    shift-right: [w142] -> _
    shift-left: w22 -> [w152]
    shift-right: [w143] -> _
    shift-left: w20 -> [w145]
    shift-right: [w105] -> _
    shift-left: w1 -> [w133]
    shift-right: [w106] -> _
    shift-left: w1 -> [w132]
    shift-right: [w110] -> _
    shift-left: w1 -> [w121]
    shift-right: [w109] -> _
    shift-left: w1 -> [w120]
    shift-right: [w103] -> _
    shift-left: w1 -> [w119]
    shift-right: [w113] -> _
    shift-left: w1 -> [w118]
    shift-right: [w104] -> _
    shift-left: w1 -> [w117]
    shift-right: [w102] -> _
    shift-left: w1 -> [w116]
    shift-right: [w108] -> _
    shift-left: w1 -> [w115]
    shift-right: [w107] -> _
    shift-left: w1 -> [w114]
    shift-right: [w95] -> w3
    shift-left: "Probe 4" -> [w195]
    shift-right: [w65] -> _
    shift-left: w1 -> [w92]
    shift-right: [w66] -> _
    shift-left: w1 -> [w91]
    shift-right: [w67] -> _
    shift-left: w1 -> [w90]
    shift-right: [w68] -> _
    shift-left: w1 -> [w89]
    i -> [w155]
    stop <- "Interrupt program" stop-if-true
    # "Ig for bias stress plots"
    # "Id for bias stress plots"
    # "Is for bias stress plots"
    # "Time axis for bias stress plots"
    # "Save bias stress curves in file."
    # "Is off"
    # "Is on"
    # "Ig off"
    # "Ig on"
    # "Is min"
    # "Is max"
    # "Ig min"
    # "Ig max"
    # "Id min"
    # "Id max"
    # "Id off"
    # "Id on"
    # "Is off"
    # "Is on"
    # "Ig off"
    # "Ig on"
    # "Is min"
    # "Is max"
    # "Ig min"
    # "Ig max"
    # "Id min"
    # "Id max"
    # "Id off"
    # "Id on"
    # "Filepath and name"
    # "Limit of command arguments (array columns). Raise if needed."
    # "Serial port data (string)"
    # "Serial port data (table)"
    # "Serial port data"
    # "For loop counter"
    # "<-----Equivalent to the 4155C \"Write\" subvi.----->"
    # "Headers"
    # "Save transfer curves in file."
    # "Filepath and name"
    # "Save time-dependent data."
    # "Use the time offset if your measurements do not start at t=0."
    # "Time for Imax, Imin, Ion, Ioff"
    # "Rest of elements of command"
    # "First element of command\n(case select)"
    n20 = Add(x=w155, y=1) -> (x+y=→"Line running":i32)
    n21 = Add(x=w160, y=1) -> (x+y=→"Total lines":i32)
    n22 = Index Array(array=w188, index=0 ("line index")) -> (element=w183:string)
    "Command running:" <- w183
    n23 = control-ref of="Interrupt scan"() -> (w207:refnum<vi>)
    n24 = Spreadsheet String To Array(delimiter (Tab)=" ", format string="%s", spreadsheet string=w183, array type (2D Dbl)=string[] []) -> (array=w181:string[])
    n25 = Delete From Array(array=w181, index=0) -> (deleted portion=w134:string, array with subset deleted=w180:string[])  [unwired: 1 in]
    n26 = call "Elapsed Time"("Reset"="Reset", "Auto Reset"="Auto Reset") -> ("Elapsed Time (s)"=w190:dbl)  [unwired: 10 in, 7 out]
    n27 = case shown="2" "Time Units" {
      tunnel: ["-sec" "-min" "-h"] -> w191
      tunnel: [w221 w225 w228] -> w161
      tunnel: w190 -> [w221 w224 w229]
      frame 0, Default {
      }
      frame 1 {
        n28 = Divide(x=w224, y=60.0) -> (x/y=w225:dbl)
      }
      frame 2 {
        n29 = Divide(x=w229, y=3600.0) -> (x/y=w228:dbl)
      }
    }
    n30 = Add(x=w161, y="Time Offset") -> (x+y=w93:dbl)
    n31 = To Long Integer(number=w93) -> (32bit integer=w94:i32)
    "Elapsed Time" <- w94
    n32 = case shown="\"sample-fpp\"" w134 {
      tunnel: w180 -> [w265 w302 w338 w354 w480 w597 w741 w865 w1030 w1062 w1135 w1180 w1223 w1262 w1294 _ _ w1478 w1603 _ w1707 w1771 w1832 w1925 w2005 w2043]
      tunnel: w217 -> [w260 w298 w336 w367 w487 w656 w749 w872 w1038 w1079 w1124 w1172 w1216 w1256 w1287 w1324 w1384 w1459 w1585 w1634 w1694 w1758 w1820 w1919 w2001 w2045]
      tunnel: w216 -> [w259 w297 w327 w366 w458 w641 w718 w843 w1006 w1080 w1125 w1173 w1217 w1257 w1288 w1329 w1386 w1484 w1609 w1638 w1713 w1777 w1838 w1931 w1959 w2049]
      tunnel: w215 -> [w258 w296 w326 w365 w457 w640 w717 w842 w1003 w1081 w1126 w1174 w1218 w1258 w1289 w1328 w1357 w1483 w1608 w1637 w1712 w1776 w1837 w1930 w1958 w2048]
      tunnel: w214 -> [w257 w295 w335 w363 w483 w617 w745 w868 w1034 w1089 w1134 w1171 w1215 w1255 w1286 w1327 w1381 w1451 w1577 w1643 w1687 w1751 w1813 w1918 w2000 w2050]
      tunnel: w213 -> [w256 w294 w334 w362 w485 w654 w747 w870 w1036 w1088 w1133 w1179 w1222 w1261 w1293 w1326 w1366 w1482 w1607 w1646 w1711 w1775 w1836 w1929 w2009 w2051]
      tunnel: w212 -> [w255 w293 w333 w360 w484 w653 w746 w869 w1035 w1087 w1132 w1178 w1221 w1260 w1292 w1325 w1367 w1460 w1586 w1645 w1695 w1759 w1821 w1920 w2002 w2053]
      tunnel: [w259 w297 w325 w366 w482 w651 w743 w867 w1032 w1080 w1125 w1173 w1217 w1257 w1288 w1329 w1386 w1452 w1559 w1636 w1688 w1752 w1814 w1872 w1961 w2049] -> w211
      tunnel: [w258 w296 w324 w365 w481 w650 w742 w866 w1031 w1081 w1126 w1174 w1218 w1258 w1289 w1328 w1356 w1461 w1560 w1635 w1696 w1760 w1822 w1871 w1960 w2047] -> w146
      tunnel: [w257 w295 w335 w363 w483 w613 w745 w868 w1034 w1082 w1127 w1171 w1215 w1255 w1286 w1327 w1381 w1451 w1577 w1643 w1687 w1751 w1813 w1918 w2000 w2050] -> w210
      tunnel: [w256 w294 w334 w362 w485 w654 w747 w870 w1036 w1088 w1133 w1179 w1222 w1261 w1293 w1326 w1366 w1482 w1607 w1646 w1711 w1775 w1836 w1929 w2009 w2051] -> w209
      tunnel: [w255 w293 w333 w360 w484 w653 w746 w869 w1035 w1087 w1132 w1178 w1221 w1260 w1292 w1325 w1367 w1460 w1586 w1645 w1695 w1759 w1821 w1920 w2002 w2053] -> w208
      tunnel: [w260 w298 w336 w367 w487 w656 w749 w872 w1038 w1079 w1124 w1172 w1216 w1256 w1287 w1324 w1384 w1459 w1585 w1634 w1694 w1758 w1820 w1919 w2001 w2045] -> w69
      tunnel: w207 -> [_ _ _ _ w489 w660 w754 w874 w1042 _ _ _ _ _ _ _ _ w1456 w1582 _ w1693 w1757 w1819 w1891 w1977 _]
      tunnel: "Gate" -> [_ _ _ _ w467 w644 w728 w852 w1017 _ _ _ _ _ _ _ _ _ _ _ _ _ _ _ _ _]
      tunnel: "Drain 2" -> [_ _ _ _ w466 w643 w727 w851 w1016 _ _ _ _ _ _ _ _ _ _ _ _ _ _ _ _ _]
      tunnel: "Panel Controls" -> [_ _ _ _ _ _ w726 w778 w1015 _ _ _ _ _ _ _ _ _ _ _ _ _ _ _ _ _]
      tunnel: w203 -> [w254 w292 w332 w359 w451 w634 w711 w836 w1001 w1086 w1131 _ w1214 w1254 w1285 w1323 w1368 w1447 w1573 w1639 w1683 w1747 w1809 w1914 w1996 w2054]
      tunnel: w202 -> [w253 w291 w331 w358 w450 w633 w710 w835 w1000 w1085 w1130 w1177 _ w1245 w1291 w1322 w1369 w1448 w1574 w1640 w1684 w1748 w1810 w1915 w1997 w2055]
      tunnel: w201 -> [w252 w290 w330 w357 w449 w632 w709 w834 w999 w1084 w1129 w1176 w1220 w1259 _ w1321 w1370 w1449 w1575 w1641 w1685 w1749 w1811 w1916 w1998 w2056]
      tunnel: w200 -> [w251 w289 w329 w356 w448 w631 w708 w833 w1002 w1083 w1128 w1175 w1219 _ w1290 w1320 w1371 w1450 w1576 w1642 w1686 w1750 w1812 w1917 w1999 w2057]
      tunnel: [w254 w292 w332 w359 w451 w634 w711 w836 w1001 w1086 w1131 w1170 w1214 w1254 w1285 w1323 w1368 w1447 w1573 w1639 w1683 w1747 w1809 w1914 w1996 w2054] -> w199
      tunnel: [w253 w291 w331 w358 w450 w633 w710 w835 w1000 w1085 w1130 w1177 w1206 w1245 w1291 w1322 w1369 w1448 w1574 w1640 w1684 w1748 w1810 w1915 w1997 w2055] -> w198
      tunnel: [w252 w290 w330 w357 w449 w632 w709 w834 w999 w1084 w1129 w1176 w1220 w1259 w1284 w1321 w1370 w1449 w1575 w1641 w1685 w1749 w1811 w1916 w1998 w2056] -> w197
      tunnel: [w251 w289 w329 w356 w448 w631 w708 w833 w1002 w1083 w1128 w1175 w1219 w1246 w1290 w1320 w1371 w1450 w1576 w1642 w1686 w1750 w1812 w1917 w1999 w2057] -> w196
      tunnel: w195 -> [w235 w270 w307 _ w389 w586 w680 w774 w970 w1059 w1107 w1154 w1190 w1229 w1268 w1304 w1334 w1434 w1539 w1618 w1654 w1722 w1785 w1851 w1936 w2014]
      tunnel: w194 -> [_ _ _ _ w442 w628 _ _ _ _ _ _ _ _ _ _ _ _ _ _ _ _ _ _ _ _]
      tunnel: [w250 w285 w322 w371 w404 w605 w698 w790 w988 w1078 w1122 w1169 w1205 w1244 w1283 w1319 w1352 w1424 w1543 w1633 w1672 w1740 w1803 w1869 w1954 w2046] -> w112
      tunnel: w193 -> [w250 w285 w322 w371 w439 w605 w698 w825 w988 w1078 w1122 w1169 w1205 w1244 w1283 w1319 w1352 w1430 w1543 w1633 w1672 w1740 w1803 w1869 w1954 w2046]
      tunnel: w93 -> [_ _ _ _ w438 w602 w696 w824 w985 _ _ _ _ _ _ _ w1350 w1439 w1555 _ w1669 w1737 w1800 w1866 w1950 _]
      tunnel: w191 -> [_ _ _ _ w435 w601 w694 w821 w984 _ _ _ _ _ _ _ w1348 w1437 w1554 _ w1668 w1736 w1799 w1865 w1951 _]
      tunnel: w94 -> [_ _ _ _ w431 _ _ w817 _ _ _ _ _ _ _ _ _ _ _ _ _ _ _ _ _ _]
      tunnel: [w249 w284 w321 w361 w408 w604 w697 w794 w987 w1077 w1121 w1168 w1204 w1243 w1282 w1318 w1351 w1409 w1557 w1632 w1671 w1739 w1802 w1868 w1953 w2052] -> w147
      tunnel: w189 -> [w249 w284 w321 w361 w434 w604 w697 w820 w987 w1077 w1121 w1168 w1204 w1243 w1282 w1318 w1351 w1411 w1557 w1632 w1671 w1739 w1802 w1868 w1953 w2052]
      tunnel: [w248 w283 w320 w370 w403 w600 w693 w789 w983 w1076 w1120 w1167 w1203 w1242 w1281 w1317 w1347 w1423 w1542 w1631 w1667 w1735 w1798 w1864 w1949 w2041] -> w111
      tunnel: w165 -> [w248 w283 w320 w370 w430 w600 w693 w816 w983 w1076 w1120 w1167 w1203 w1242 w1281 w1317 w1347 w1429 w1542 w1631 w1667 w1735 w1798 w1864 w1949 w2041]
      tunnel: [w247 w282 w319 w355 w423 w599 w692 w809 w982 w1075 w1119 w1166 w1202 w1241 w1280 w1316 w1346 w1436 w1553 w1630 w1666 w1734 w1797 w1863 w1948 w2040] -> w142
      tunnel: w152 -> [w247 w282 w319 w355 w423 w599 w692 w809 w982 w1075 w1119 w1166 w1202 w1241 w1280 w1316 w1346 w1436 w1553 w1630 w1666 w1734 w1797 w1863 w1948 w2039]
      tunnel: [w246 w281 w318 w364 w422 w598 w691 w808 w981 w1074 w1118 w1165 w1201 w1240 w1279 w1315 w1345 w1435 w1552 w1629 w1665 w1733 w1796 w1862 w1947 w2025] -> w143
      tunnel: w145 -> [w246 w281 w318 w364 w422 w598 w691 w808 w981 w1074 w1118 w1165 w1201 w1240 w1279 w1315 w1345 w1435 w1552 w1629 w1665 w1733 w1796 w1862 w1947 w2025]
      tunnel: [w244 w279 w316 w376 w397 w595 w689 w783 w979 w1072 w1117 w1164 w1199 w1238 w1277 w1313 w1343 w1417 w1551 w1628 w1664 w1732 w1794 w1861 w1946 w2024] -> w105
      tunnel: w133 -> [w244 w279 w316 w376 w421 w595 w689 w807 w979 w1072 w1117 w1164 w1199 w1238 w1277 w1313 w1343 w1417 w1551 w1628 w1664 w1732 w1794 w1861 w1946 w2024]
      tunnel: [w245 w280 w317 w377 w398 w596 w690 w784 w980 w1073 w1116 w1163 w1200 w1239 w1278 w1314 w1344 w1418 w1550 w1627 w1663 w1731 w1795 w1860 w1945 w2023] -> w106
      tunnel: w132 -> [w245 w280 w317 w377 w420 w596 w690 w806 w980 w1073 w1116 w1163 w1200 w1239 w1278 w1314 w1344 w1418 w1550 w1627 w1663 w1731 w1795 w1860 w1945 w2023]
      tunnel: [w237 w272 w309 w369 w402 w592 w687 w788 w977 w1065 w1114 w1161 w1197 w1236 w1275 w1311 w1336 w1422 w1541 w1626 w1656 w1724 w1787 w1853 w1940 w2016] -> w110
      tunnel: w121 -> [w237 w272 w309 w369 w416 w592 w687 w802 w977 w1065 w1114 w1161 w1197 w1236 w1275 w1311 w1336 w1428 w1541 w1626 w1656 w1724 w1787 w1853 w1940 w2016]
      tunnel: [w236 w271 w308 w368 w401 w593 w688 w787 w978 w1064 w1115 w1162 w1198 w1237 w1276 w1312 w1335 w1421 w1540 w1625 w1655 w1723 w1786 w1852 w1939 w2015] -> w109
      tunnel: w120 -> [w236 w271 w308 w368 w415 w593 w688 w801 w978 w1064 w1115 w1162 w1198 w1237 w1276 w1312 w1335 w1427 w1540 w1625 w1655 w1723 w1786 w1852 w1939 w2015]
      tunnel: [w239 w274 w311 w373 w407 w591 w685 w793 w975 w1070 w1112 w1159 w1195 w1234 w1273 w1309 w1338 w1426 w1545 w1620 w1658 w1726 w1789 w1855 w1938 w2020] -> w103
      tunnel: w119 -> [w239 w274 w311 w373 w414 w591 w685 w800 w975 w1070 w1112 w1159 w1195 w1234 w1273 w1309 w1338 w1432 w1545 w1620 w1658 w1726 w1789 w1855 w1938 w2020]
      tunnel: [w238 w273 w310 w372 w405 w594 w686 w791 w976 w1071 w1113 w1160 w1196 w1235 w1274 w1310 w1337 w1425 w1544 w1619 w1657 w1725 w1788 w1854 w1937 w2019] -> w113
      tunnel: w118 -> [w238 w273 w310 w372 w413 w594 w686 w799 w976 w1071 w1113 w1160 w1196 w1235 w1274 w1310 w1337 w1431 w1544 w1619 w1657 w1725 w1788 w1854 w1937 w2019]
      tunnel: [w241 w276 w313 w375 w396 w590 w683 w782 w973 w1068 w1110 w1157 w1193 w1232 w1271 w1307 w1340 w1416 w1547 w1622 w1660 w1728 w1791 w1857 w1942 w2022] -> w104
      tunnel: w117 -> [w241 w276 w313 w375 w412 w590 w683 w798 w973 w1068 w1110 w1157 w1193 w1232 w1271 w1307 w1340 w1416 w1547 w1622 w1660 w1728 w1791 w1857 w1942 w2022]
      tunnel: [w240 w275 w312 w374 w395 w589 w684 w781 w974 w1069 w1111 w1158 w1194 w1233 w1272 w1308 w1339 w1415 w1546 w1621 w1659 w1727 w1790 w1856 w1941 w2021] -> w102
      tunnel: w116 -> [w240 w275 w312 w374 w411 w589 w684 w797 w974 w1069 w1111 w1158 w1194 w1233 w1272 w1308 w1339 w1415 w1546 w1621 w1659 w1727 w1790 w1856 w1941 w2021]
      tunnel: [w243 w278 w315 w379 w400 w588 w681 w786 w971 w1066 w1108 w1155 w1191 w1230 w1269 w1305 w1342 w1420 w1549 w1624 w1662 w1730 w1793 w1859 w1944 w2018] -> w108
      tunnel: w115 -> [w243 w278 w315 w379 w410 w588 w681 w796 w971 w1066 w1108 w1155 w1191 w1230 w1269 w1305 w1342 w1420 w1549 w1624 w1662 w1730 w1793 w1859 w1944 w2018]
      tunnel: [w242 w277 w314 w378 w399 w587 w682 w785 w972 w1067 w1109 w1156 w1192 w1231 w1270 w1306 w1341 w1419 w1548 w1623 w1661 w1729 w1792 w1858 w1943 w2017] -> w107
      tunnel: w114 -> [w242 w277 w314 w378 w409 w587 w682 w795 w972 w1067 w1109 w1156 w1192 w1231 w1270 w1306 w1341 w1419 w1548 w1623 w1661 w1729 w1792 w1858 w1943 w2017]
      tunnel: [w235 w270 w307 w345 w389 w586 w680 w774 w970 w1059 w1107 w1154 w1190 w1229 w1268 w1304 w1334 w1434 w1539 w1618 w1654 w1722 w1785 w1851 w1936 w2014] -> w95
      tunnel: w93 -> [_ _ _ _ _ _ _ _ _ _ _ _ _ _ _ _ _ w1405 _ _ _ _ _ _ _ _]
      tunnel: [w234 w269 w306 w344 w388 w585 w679 w773 w969 w1058 w1106 w1153 w1189 w1228 w1267 w1303 w1333 w1396 w1538 w1617 w1653 w1721 w1784 w1850 w1935 w2013] -> w65
      tunnel: [w233 w268 w305 w343 w387 w584 w678 w772 w968 w1057 w1105 w1152 w1188 w1227 w1266 w1302 w1332 w1393 w1537 w1616 w1652 w1720 w1783 w1849 w1934 w2012] -> w66
      tunnel: [w232 w267 w304 w342 w386 w583 w677 w771 w967 w1056 w1104 w1151 w1187 w1226 w1265 w1301 w1331 w1394 w1536 w1615 w1651 w1719 w1782 w1848 w1933 w2011] -> w67
      tunnel: [w231 w266 w303 w341 w385 w582 w676 w770 w966 w1055 w1103 w1150 w1186 w1225 w1264 w1300 w1330 w1395 w1535 w1614 w1650 w1718 w1781 w1847 w1932 w2010] -> w68
      tunnel: w92 -> [w234 w269 w306 w344 w388 w585 w679 w773 w969 w1058 w1106 w1153 w1189 w1228 w1267 w1303 w1333 w1400 w1538 w1617 w1653 w1721 w1784 w1850 w1935 w2013]
      tunnel: w91 -> [w233 w268 w305 w343 w387 w584 w678 w772 w968 w1057 w1105 w1152 w1188 w1227 w1266 w1302 w1332 w1399 w1537 w1616 w1652 w1720 w1783 w1849 w1934 w2012]
      tunnel: w90 -> [w232 w267 w304 w342 w386 w583 w677 w771 w967 w1056 w1104 w1151 w1187 w1226 w1265 w1301 w1331 w1398 w1536 w1615 w1651 w1719 w1782 w1848 w1933 w2011]
      tunnel: w89 -> [w231 w266 w303 w341 w385 w582 w676 w770 w966 w1055 w1103 w1150 w1186 w1225 w1264 w1300 w1330 w1397 w1535 w1614 w1650 w1718 w1781 w1847 w1932 w2010]
      tunnel: "Standby" -> [_ _ _ _ w384 w581 _ w769 _ _ _ _ _ _ _ _ _ w1391 w1534 _ _ _ _ w1846 _ _]
      frame "wait" {
        n33 = Index Array(array=w265, index=0 ("Index")) -> (element=w263:string)
        n34 = Decimal String To Number(string=w263, default (0L)=u32 0) -> (number=w262:u32)  [unwired: 1 in, 1 out]
        n35 = Wait (ms)(milliseconds to wait=w262) -> ()  [unwired: 1 out]
      }
      frame "wait-min" {
        n36 = Index Array(array=w302, index=0 ("Index")) -> (element=w300:string)
        n37 = Decimal String To Number(string=w300, default (0L)=u32 0) -> (number=w288:u32)  [unwired: 1 in, 1 out]
        n38 = Multiply(x=w288, y=u32 60000) -> (x*y=w287:u32)
        n39 = Wait (ms)(milliseconds to wait=w287) -> ()  [unwired: 1 out]
      }
      frame "standby" {
        n40 = Index Array(array=w338, index=0 ("Index")) -> (element=w328:string)
        n41 = case shown="\"off\", Default" w328 {
          tunnel: [":PAGE:SCON:STAN 0" ":PAGE:SCON:STAN 1"] -> w323
          frame "off", Default {
          }
          frame "on" {
          }
        }
        n42 = VISA Write(VISA resource name=w327, write buffer=w323, error in (no error)=w326) -> (VISA resource name out=w325:refnum<visa-resource-name>, error out=w324:errorcluster)  [unwired: 1 out]
      }
      frame "Probe4" {
        n43 = Delete From Array(array=w354, index=0) -> (deleted portion=w348:string, array with subset deleted=w351:string[])  [unwired: 1 in]
        n44 = Equal?(x=w348, y="ON") -> (x = y?=w346:bool)
        n45 = Delete From Array(array=w351, index=0) -> (deleted portion=w350:string)  [unwired: 1 in, 1 out]
        n46 = Fract/Exp String To Number(string=w350) -> (number=w347:dbl)  [unwired: 3 in, 1 out]
        n47 = Bundle(w346, w347) -> (w345:cluster{bool, dbl})  [unwired: 1 in]
      }
      frame "transfer" {
        n48 = local read "Transfer/Output - Gate"() -> (w383:u32)
        n49 = Delete From Array(array=w480, index=0 ("Index")) -> (deleted portion=w478:string, array with subset deleted=w477:string[])  [unwired: 1 in]
        n50 = Bundle By Name(cluster=w442, "Emergency Stop"=w489) -> (w443:T2)
        n51 = Number To Decimal String(number=w438) -> (decimal integer string=w437:string)  [unwired: 1 in]
        n52 = case shown="\"d\", Default" w478 {
          tunnel: [w574 w575] -> w476
          frame "s" {
            w574 = u16 0 items=["Single", "Double"] ("sweep mode")
          }
          frame "d", Default {
            w575 = u16 1 items=["Single", "Double"] ("sweep mode")
          }
        }
        n53 = Fract/Exp String To Number(string=w477) -> (number=w462:dbl[])  [unwired: 3 in, 1 out]
        n54 = Concatenate Strings(w487, "-transfer-" ("Prefix"), w437, w435, ".txt" ("Suffix (transfer)")) -> (w488:string)
        n55 = VISA Write(VISA resource name=w458, write buffer=":PAGE:CHAN:MODE SWE;" ("write buffer (\"\")"), error in (no error)=w457) -> (VISA resource name out=w455:refnum<visa-resource-name>, error out=w456:errorcluster)  [unwired: 1 out]
        n56 = local read "Plot transfer curve extrema vs time"() -> (w390:bool)
        n57 = String To Path(string=w488) -> (path=w486:path)
        n58 = Index Array(array=w462, index #1=0 ("Index")) -> (element #1=w475:dbl, element #2=w474:dbl, element #3=w473:dbl)  [unwired: 2 in]
        n59 = Delete From Array(array=w462, length=3 ("Length"), index=0 ("Index")) -> (array with subset deleted=w460:dbl[])  [unwired: 1 out]
        n60 = local read "Transfer/Output - Drain"() -> (w380:u32)
        n61 = local read "Transfer/Output - Source/Common"() -> (w382:u32)
        n62 = case shown="True" w390 {
          tunnel: w434 -> [w491 w494]
          tunnel: w431 -> [_ w493]
          tunnel: [w491 w492] -> w408
          frame False {
          }
          frame True {
            n63 = Build Array (concatenate)(w494, w493) -> (w492:i32[])
          }
        }
        n64 = local read "Transfer/Output - Probe 4"() -> (w381:u32)
        n65 = Bundle By Name(cluster=w467, "Gate Start"=w475, "Gate Stop"=w474, "Gate Step (linear only)"=w473, "Gate Compliance"=w484, "Range mode"=w451, "Range"=w450) -> (w452:T6)
        n66 = Index Array(array=w460, index #1=0 ("Index")) -> (element #1=w470:dbl, element #2=w469:dbl, element #3=w468:dbl)  [unwired: 2 in]
        n67 = call <vilib>:"compatOverwrite.vi"("overwrite (F)"=TRUE) -> ("overwrite?"=w441:T8)
        n68 = Bundle By Name(cluster=w466, "Drain Start"=w470, "Drain Stop"=w469, "Drain Step"=w468, "Drain Compliance"=w485, "Range mode"=w449, "Range"=w448) -> (w453:T7)
        n69 = call "4155C Transfer v2.0.vi"("VISA resource name in"=w455, "Source/Common"=w382, 2:"Gate"=w452, 3:"Drain"=w453, 4:"Drain"=w380, "Timings"=w483, "error in (no error)"=w456, 7:"Probe 4"=w389, 8:"Gate"=w383, 9:"Probe 4"=w381, "sweep mode"=w476, "Panel Controls"=w443, "Standby"=w384) -> ("VG"=w440:dbl[], "Outparams"=w447:T9, "VISA Resource Name out"=w482:refnum<visa-resource-name>, "IS"=w418:dbl[], "ID"=w419:dbl[], "IG"=w417:dbl[], "error out"=w432:errorcluster, "Probe 4"=w444:dbl[])  [unwired: 7 in]
        n70 = Unbundle By Name(w447) -> ("V2 Step"=w446:dbl, "V2 Start"=w445:dbl, "Number of points"=w406:i32)
        n71 = call "4155C Split array.vi"("Number of VAR2 steps"=w406, "Y2 data in"=w419, "X data in"=w440, "Y1 data in"=w418, "Y3 data in"=w417, "error in (no error)"=w432) -> ("Array of clusters"=w433:cluster{"Y data in":dbl[], "X data in":dbl[]}[], "error out"=w394:errorcluster)  [unwired: 1 in]
        n72 = case shown="True" "Plot transfer curve extrema vs time" {
          tunnel: w439 -> [w497 w573]
          tunnel: w430 -> [w498 w568]
          tunnel: w421 -> [w504 w564]
          tunnel: w420 -> [w505 w563]
          tunnel: w419 -> [_ w560]
          tunnel: w418 -> [_ w558]
          tunnel: w417 -> [_ w557]
          tunnel: w416 -> [w499 w553]
          tunnel: w415 -> [w501 w552]
          tunnel: w414 -> [w495 w549]
          tunnel: w413 -> [w496 w548]
          tunnel: w412 -> [w503 w545]
          tunnel: w411 -> [w502 w544]
          tunnel: w410 -> [w507 w541]
          tunnel: w409 -> [w506 w540]
          tunnel: w408 -> [_ w533]
          tunnel: [w495 w528] -> w407
          tunnel: w406 -> [_ w527]
          tunnel: [w496 w526] -> w405
          tunnel: [w497 w525] -> w404
          tunnel: [w498 w524] -> w403
          tunnel: [w499 w523] -> w402
          tunnel: [w501 w522] -> w401
          tunnel: [w507 w521] -> w400
          tunnel: [w506 w520] -> w399
          tunnel: [w505 w519] -> w398
          tunnel: [w504 w518] -> w397
          tunnel: [w503 w517] -> w396
          tunnel: [w502 w516] -> w395
          tunnel: w394 -> [w500 w515]
          tunnel: [w500 w511] -> w393
          frame False {
          }
          frame True {
            # "Adjusts graph colors."
            # "Adjusts graph colors."
            # "Ion will be the middle element of the array. The calculation of the index is done only once, since Is, Id, and Ig have the same dimensions."
            # "abs(Ig)"
            # "abs(Is)"
            # "Y1: Is\nY2: Id\nY3: Ig"
            # "abs(Id)"
            # "Adjusts graph colors."
            # "Adjusts graph colors."
            # "Adjusts graph colors."
            n73 = Absolute Value(x=w558) -> (abs(x)=w543:dbl[])
            n74 = Absolute Value(x=w560) -> (abs(x)=w559:dbl[])
            n75 = Absolute Value(x=w557) -> (abs(x)=w546:dbl[])
            n76 = Array Size(array=w559) -> (size(s)=w567:i32)
            n77 = Divide(x=w567, y=2) -> (x/y=w510:dbl)
            n78 = Subtract(x=w510, y=1) -> (x-y=w509:dbl)
            n79 = Array Max & Min(array=w543) -> (max value=w550:dbl, min value=w551:dbl)  [unwired: 2 out]
            n80 = Array Max & Min(array=w559) -> (max value=w572:dbl, min value=w556:dbl)  [unwired: 2 out]
            n81 = Array Max & Min(array=w546) -> (max value=w555:dbl, min value=w554:dbl)  [unwired: 2 out]
            n82 = Index Array(array=w543, index=w509) -> (element=w534:dbl)
            n83 = Index Array(array=w543, index=0) -> (element=w535:dbl)
            n84 = Index Array(array=w559, index=w509) -> (element=w536:dbl)
            n85 = Index Array(array=w559, index=0) -> (element=w537:dbl)
            n86 = Index Array(array=w546, index=w509) -> (element=w539:dbl)
            n87 = Index Array(array=w546, index=0) -> (element=w538:dbl)
            n88 = local write "Ig max"(w555) -> ()
            n89 = local write "Ig min"(w554) -> ()
            n90 = local write "Is max"(w550) -> ()
            n91 = local write "Is min"(w551) -> ()
            n92 = local write "Id max"(w572) -> ()
            n93 = local write "Id min"(w556) -> ()
            n94 = Build Array (concatenate)(w549, w550) -> (w528:dbl[])
            n95 = Build Array (concatenate)(w548, w551) -> (w526:dbl[])
            n96 = local write "Is off"(w535) -> ()
            n97 = local write "Is on"(w534) -> ()
            n98 = Build Array (concatenate)(w573, w572) -> (w525:dbl[])
            n99 = Build Array (concatenate)(w568, w556) -> (w524:dbl[])
            n100 = Build Array (concatenate)(w553, w555) -> (w523:dbl[])
            n101 = Build Array (concatenate)(w552, w554) -> (w522:dbl[])
            n102 = Build Array (concatenate)(w541, w534) -> (w521:dbl[])
            n103 = Build Array (concatenate)(w540, w535) -> (w520:dbl[])
            n104 = Build Array (concatenate)(w563, w536) -> (w519:dbl[])
            n105 = Build Array (concatenate)(w564, w537) -> (w518:dbl[])
            n106 = Build Array (concatenate)(w545, w539) -> (w517:dbl[])
            n107 = Build Array (concatenate)(w544, w538) -> (w516:dbl[])
            n108 = local write "Ig off"(w538) -> ()
            n109 = local write "Ig on"(w539) -> ()
            n110 = local write "Id off"(w537) -> ()
            n111 = local write "Id on"(w536) -> ()
            n112 = control-ref of="Imax vs time"() -> (w562:refnum<vi>)
            n113 = control-ref of="Imin vs time"() -> (w561:refnum<vi>)
            n114 = control-ref of="Ion vs time"() -> (w530:refnum<vi>)
            n115 = control-ref of="Ioff vs time"() -> (w529:refnum<vi>)
            n116 = control-ref of="I vs Vg"() -> (w571:refnum<vi>)
            n117 = call "4155C Split array.vi"("Number of VAR2 steps"=w527, "Y2 data in"=w519, "X data in"=w533, "Y1 data in"=w521, "Y3 data in"=w517, "error in (no error)"=w515) -> ("Array of clusters"=w531:cluster{"Y data in":dbl[], "X data in":dbl[]}[], "error out"=w514:errorcluster)  [unwired: 1 in]
            n118 = call "4155C Split array.vi"("Number of VAR2 steps"=w527, "Y2 data in"=w518, "X data in"=w533, "Y1 data in"=w520, "Y3 data in"=w516, "error in (no error)"=w514) -> ("Array of clusters"=w532:cluster{"Y data in":dbl[], "X data in":dbl[]}[], "error out"=w513:errorcluster)  [unwired: 1 in]
            n119 = call "4155C Split array.vi"("Number of VAR2 steps"=w527, "Y2 data in"=w525, "X data in"=w533, "Y1 data in"=w528, "Y3 data in"=w523, "error in (no error)"=w513) -> ("Array of clusters"=w570:cluster{"Y data in":dbl[], "X data in":dbl[]}[], "error out"=w512:errorcluster)  [unwired: 1 in]
            n120 = call "4155C Split array.vi"("Number of VAR2 steps"=w527, "Y2 data in"=w524, "X data in"=w533, "Y1 data in"=w526, "Y3 data in"=w522, "error in (no error)"=w512) -> ("Array of clusters"=w569:cluster{"Y data in":dbl[], "X data in":dbl[]}[], "error out"=w511:errorcluster)  [unwired: 1 in]
            n121 = call "4155C Config Chart Colours.vi"("Numeric"=w527, "XY Graph 2"=w562) -> ()  [unwired: 6 in]
            n122 = call "4155C Config Chart Colours.vi"("Numeric"=w527, "XY Graph 2"=w561) -> ()  [unwired: 6 in]
            n123 = call "4155C Config Chart Colours.vi"("Numeric"=w527, "XY Graph 2"=w530) -> ()  [unwired: 6 in]
            n124 = call "4155C Config Chart Colours.vi"("Numeric"=w527, "XY Graph 2"=w529) -> ()  [unwired: 6 in]
            n125 = call "4155C Config Chart Colours.vi"("Numeric"=w527, "XY Graph 2"=w571) -> ()  [unwired: 6 in]
            n126 = local write "Imax vs time"(w570) -> ()
            n127 = local write "Imin vs time"(w569) -> ()
            n128 = local write "Ion vs time"(w531) -> ()
            n129 = local write "Ioff vs time"(w532) -> ()
          }
        }
        n130 = local write "I vs Vg"(w433) -> ()
        n131 = Open/Create/Replace File(file path (use dialog)=w486, error in=w393, operation (0:open)=w441) -> (refnum out=w428:refnum<file>, error out=w426:errorcluster)  [unwired: 3 in, 1 out]
        n132 = call "4155C Make Big 2d array.vi"("1D Var1"=w440, "1d IS"=w418, "1d ID"=w419, "1d IG"=w417, "1d SMU4"=w444, "SMU4"=w389, "VAR2 START"=w445, "Number of VAR2 steps"=w406, "VAR2 STEP"=w446, "VAR1 Name"="Vg", "Decimal places in header"=i8 1, "VAR2 Name"="Vd") -> ("Header array"=w429:string[], "Data array"=w427:dbl[][])  [unwired: 14 in]
        n133 = call "4155C Write array to file.vi"("Byte Stream File Refnum"=w428, "Header"=w429, "Data Array"=w427, "error in (no error)"=w426) -> ("dup refnum"=w425:refnum<file>, "error out"=w424:errorcluster)  [unwired: 1 in]
        n134 = Close File(refnum=w425, error in=w424) -> (error out=w481:errorcluster)  [unwired: 1 out]
      }
      frame "pulsedstressV" {
        w611 = 0
        n135 = local read "Pulsed Stress V - Drain"() -> (w580:u32)
        n136 = local read "Pulsed Stress V - Gate"() -> (w577:u32)
        n137 = local read "Pulsed Stress V - Probe 4"() -> (w579:u32)
        n138 = local read "Pulsed Stress V - Source/Common"() -> (w576:u32)
        n139 = local read "Pulsed Stress V - Vextra"() -> (w578:u32)
        n140 = Number To Decimal String(number=w602) -> (decimal integer string=w657:string)  [unwired: 1 in]
        n141 = Delete From Array(array=w597, index=0 ("Index")) -> (deleted portion=w648:string, array with subset deleted=w647:string[])  [unwired: 1 in]
        n142 = Bundle By Name(cluster=w628, "Emergency Stop"=w660) -> (w629:T2)
        n143 = VISA Write(VISA resource name=w641, write buffer=":PAGE:CHAN:MODE SWE;" ("write buffer (\"\")"), error in (no error)=w640) -> (VISA resource name out=w638:refnum<visa-resource-name>, error out=w639:errorcluster)  [unwired: 1 out]
        n144 = Concatenate Strings(w656, "-pulsedstressV-" ("Substring"), w657, w601, ".txt" ("Substring")) -> (w659:string)
        n145 = case shown="\"d\", Default" w648 {
          tunnel: [w669 w670] -> w646
          frame "s" {
            w669 = u16 0 items=["Single", "Double"] ("sweep mode")
          }
          frame "d", Default {
            w670 = u16 1 items=["Single", "Double"] ("sweep mode")
          }
        }
        n146 = Fract/Exp String To Number(string=w647) -> (number=w642:dbl[])  [unwired: 3 in, 1 out]
        n147 = String To Path(string=w659) -> (path=w655:path)
        n148 = Index Array(array=w642, index #1=0 ("Index")) -> (element #1=w620:dbl, element #2=w619:dbl, element #3=w616:dbl, element #4=w615:dbl, element #5=w614:dbl, element #6=w618:dbl)  [unwired: 5 in]
        n149 = Bundle By Name(cluster=w617, "Pulse period"=w615, "Base voltage"=w616, "Pulse width"=w614) -> (w613:T4)
        n150 = Unbundle By Name(w613) -> ("Pulse period"=w621:dbl)
        n151 = Bundle By Name(cluster=w644, "Gate Start"=w619, "Gate Stop"=w620, "Gate Step (linear only)"=0, "Gate Compliance"=w653, "Range mode"=w634, "Range"=w633) -> (w635:T6)
        n152 = call <vilib>:"compatOverwrite.vi"("overwrite (F)"=TRUE) -> ("overwrite?"=w606:T8)
        n153 = Bundle By Name(cluster=w643, "Drain Start"=w618, "Drain Stop"=w611, "Drain Step"=w611, "Drain Compliance"=w654, "Range mode"=w632, "Range"=w631) -> (w636:T7)
        n154 = call "4155C PulsedStressV v2.0.vi"("VISA resource name in"=w638, "Gate"=w635, "Pulsed Stress V - Source/Common"=w576, "Drain"=w636, "Timings"=w613, "error in (no error)"=w639, "sweep mode"=w646, "Probe 4"=w586, "Pulsed Stress V - Drain"=w580, "Pulsed Stress V - Gate"=w577, "Panel Controls"=w629, "Standby"=w581, "Pulsed Stress V - Probe 4"=w579, "Pulsed Stress V - Vextra"=w578) -> ("Outparams"=w630:T9, "VISA Resource Name out"=w651:refnum<visa-resource-name>, "ID"=w609:dbl[], "IG"=w607:dbl[], "error out"=w652:errorcluster)  [unwired: 1 in]
        n155 = Unbundle By Name(w630) -> ("Number of points"=w608:i32)  [unwired: 2 out]
        n156 = for {
          N: w608 -> [_]
          tunnel: [w666] -> w610 mode=indexing
          tunnel: w621 -> [w668]
          i -> [w667]
          n157 = Multiply(x=w668, y=w667) -> (x*y=w666:dbl)
        }
        n158 = Insert Into Array(array=dbl[][] [] ("Input Array"), new element=w610) -> (w622:dbl[][])  [unwired: 2 in]
        n159 = Insert Into Array(array=w622, new element=w609) -> (w627:dbl[][])  [unwired: 2 in]
        n160 = Insert Into Array(array=w627, new element=w607) -> (w626:dbl[][])  [unwired: 2 in]
        n161 = Transpose 2D Array(2D array=w626) -> (transposed array=w625:dbl[][])
        n162 = Open/Create/Replace File(file path (use dialog)=w655, error in=w652, operation (0:open)=w606) -> (refnum out=w663:refnum<file>, error out=w664:errorcluster)  [unwired: 3 in, 1 out]
        n163 = call "4155C Write array to file.vi"("Byte Stream File Refnum"=w663, "Header"=string[] ["Time /s", "Id /A", "Ig /A"], "Data Array"=w625, "error in (no error)"=w664) -> ("dup refnum"=w661:refnum<file>, "error out"=w662:errorcluster)  [unwired: 1 in]
        n164 = Close File(refnum=w661, error in=w662) -> (error out=w650:errorcluster)  [unwired: 1 out]
      }
      frame "transfer-fpp" {
        n165 = local read "FPP - Source"() -> (w675:u32)
        n166 = local read "FPP - Drain"() -> (w673:u32)
        n167 = local read "FPP - Gate"() -> (w674:u32)
        n168 = local read "FPP - Probe 1"() -> (w671:u32)
        n169 = local read "FPP - Probe 2"() -> (w672:u32)
        n170 = Number To Decimal String(number=w696) -> (decimal integer string=w750:string)  [unwired: 1 in]
        n171 = Bundle By Name(cluster=w726, "Emergency Stop"=w754) -> (w762:T1)
        n172 = Delete From Array(array=w741, index=0 ("Index")) -> (deleted portion=w739:string, array with subset deleted=w738:string[])  [unwired: 1 in]
        n173 = Concatenate Strings(w749, "-transferfpp-" ("Substring"), w750, w694, ".txt" ("Substring")) -> (w752:string)
        n174 = VISA Write(VISA resource name=w718, write buffer=":PAGE:CHAN:MODE SWE;" ("write buffer (\"\")"), error in (no error)=w717) -> (VISA resource name out=w715:refnum<visa-resource-name>, error out=w716:errorcluster)  [unwired: 1 out]
        n175 = case shown="\"d\", Default" w739 {
          tunnel: [w763 w764] -> w737
          frame "s" {
            w763 = u16 0 items=["Single", "Double"] ("sweep mode")
          }
          frame "d", Default {
            w764 = u16 1 items=["Single", "Double"] ("sweep mode")
          }
        }
        n176 = Fract/Exp String To Number(string=w738) -> (number=w722:dbl[])  [unwired: 3 in, 1 out]
        n177 = String To Path(string=w752) -> (path=w748:path)
        n178 = Index Array(array=w722, index #1=0 ("Index")) -> (element #1=w736:dbl, element #2=w735:dbl, element #3=w734:dbl)  [unwired: 2 in]
        n179 = Delete From Array(array=w722, length=3 ("Length"), index=0 ("Index")) -> (array with subset deleted=w720:dbl[])  [unwired: 1 out]
        n180 = Bundle By Name(cluster=w728, "Gate Start"=w736, "Gate Stop"=w735, "Gate Step (linear only)"=w734, "Gate Compliance"=w746, "Range mode"=w711, "Range"=w710) -> (w712:T6)
        n181 = Index Array(array=w720, index #1=0 ("Index")) -> (element #1=w731:dbl, element #2=w730:dbl, element #3=w729:dbl)  [unwired: 2 in]
        n182 = call <vilib>:"compatOverwrite.vi"("overwrite (F)"=TRUE) -> ("overwrite?"=w699:T8)
        n183 = Bundle By Name(cluster=w727, "Drain Start"=w731, "Drain Stop"=w730, "Drain Step"=w729, "Drain Compliance"=w747, "Range mode"=w709, "Range"=w708) -> (w713:T7)
        n184 = call "4155C Transfer-FPP v2.0.vi"("VISA resource name in"=w715, "FPP - Source"=w675, "Gate"=w712, "Drain"=w713, "FPP - Drain"=w673, "Timings"=w745, "error in (no error)"=w716, "FPP - Gate"=w674, "FPP - Probe 1"=w671, "sweep mode"=w737, "FPP - Probe 2"=w672, "Panel Controls"=w762) -> ("VG"=w753:dbl[], "Outparams"=w707:T9, "VISA Resource Name out"=w743:refnum<visa-resource-name>, "Vprobe2"=w703:dbl[], "ID"=w702:dbl[], "IG"=w701:dbl[], "Vprobe1"=w700:dbl[], "error out"=w744:errorcluster)  [unwired: 8 in]
        n185 = Unbundle By Name(w707) -> ("V2 Step"=w706:dbl, "V2 Start"=w705:dbl, "Number of points"=w704:i32)
        n186 = Open/Create/Replace File(file path (use dialog)=w748, error in=w744, operation (0:open)=w699) -> (refnum out=w759:refnum<file>, error out=w760:errorcluster)  [unwired: 3 in, 1 out]
        n187 = call "4155C Make Big 2d array FPP.vi"("1D Var1"=w753, "1d ID"=w702, "1d Vp2"=w703, "1d IG"=w701, "1d Vp1"=w700, "VAR2 START"=w705, "Number of VAR2 steps"=w704, "VAR2 STEP"=w706, "VAR1 Name"="Vg", "Decimal places in header"=i8 1, "VAR2 Name"="Vd") -> ("Header array"=w755:string[], "Data array"=w756:dbl[][])  [unwired: 15 in]
        n188 = call "4155C Write array to file.vi"("Byte Stream File Refnum"=w759, "Header"=w755, "Data Array"=w756, "error in (no error)"=w760) -> ("dup refnum"=w757:refnum<file>, "error out"=w758:errorcluster)  [unwired: 1 in]
        n189 = Close File(refnum=w757, error in=w758) -> (error out=w742:errorcluster)  [unwired: 1 out]
      }
      frame "output" {
        n190 = local read "Transfer/Output - Drain"() -> (w766:u32)
        n191 = local read "Transfer/Output - Source/Common"() -> (w765:u32)
        n192 = local read "Transfer/Output - Gate"() -> (w767:u32)
        n193 = Delete From Array(array=w865, index=0 ("Index")) -> (deleted portion=w863:string, array with subset deleted=w862:string[])  [unwired: 1 in]
        n194 = Bundle By Name(cluster=w778, "Emergency Stop"=w874) -> (w828:T1)
        n195 = Number To Decimal String(number=w824) -> (decimal integer string=w823:string)  [unwired: 1 in]
        n196 = case shown="\"d\", Default" w863 {
          tunnel: [w959 w960] -> w861
          frame "s" {
            w959 = u16 0 items=["Single", "Double"] ("sweep mode")
          }
          frame "d", Default {
            w960 = u16 1 items=["Single", "Double"] ("sweep mode")
          }
        }
        n197 = Fract/Exp String To Number(string=w862) -> (number=w847:dbl[])  [unwired: 3 in, 1 out]
        n198 = Concatenate Strings(w872, "-output-" ("Substring"), w823, w821, ".txt" ("Suffix (transfer)")) -> (w873:string)
        n199 = VISA Write(VISA resource name=w843, write buffer=":PAGE:CHAN:MODE SWE;" ("write buffer (\"\")"), error in (no error)=w842) -> (VISA resource name out=w840:refnum<visa-resource-name>, error out=w841:errorcluster)  [unwired: 1 out]
        n200 = String To Path(string=w873) -> (path=w871:path)
        n201 = Index Array(array=w847, index #1=0 ("Index")) -> (element #1=w860:dbl, element #2=w859:dbl, element #3=w858:dbl)  [unwired: 2 in]
        n202 = Delete From Array(array=w847, length=3 ("Length"), index=0 ("Index")) -> (array with subset deleted=w845:dbl[])  [unwired: 1 out]
        n203 = local read "Plot output curve extrema vs time"() -> (w775:bool)
        n204 = local read "Transfer/Output - Probe 4"() -> (w768:u32)
        n205 = Bundle By Name(cluster=w852, "Gate Start"=w860, "Gate Stop"=w859, "Gate Step (linear only)"=w858, "Gate Compliance"=w869, "Range mode"=w836, "Range"=w835) -> (w837:T6)
        n206 = case shown="True" w775 {
          tunnel: w820 -> [w876 w879]
          tunnel: w817 -> [_ w878]
          tunnel: [w876 w877] -> w794
          frame False {
          }
          frame True {
            n207 = Build Array (concatenate)(w879, w878) -> (w877:i32[])
          }
        }
        n208 = Index Array(array=w845, index #1=0 ("Index")) -> (element #1=w855:dbl, element #2=w854:dbl, element #3=w853:dbl)  [unwired: 2 in]
        n209 = call <vilib>:"compatOverwrite.vi"("overwrite (F)"=TRUE) -> ("overwrite?"=w827:T8)
        n210 = Bundle By Name(cluster=w851, "Drain Start"=w855, "Drain Stop"=w854, "Drain Step"=w853, "Drain Compliance"=w870, "Range mode"=w834, "Range"=w833) -> (w838:T7)
        n211 = call "4155C Output v2.0.vi"("VISA resource name in"=w840, "Source/Common"=w765, 2:"Gate"=w837, 3:"Drain"=w838, 4:"Drain"=w766, "Timings"=w868, "error in (no error)"=w841, 7:"Probe 4"=w774, 8:"Gate"=w767, 9:"Probe 4"=w768, "sweep mode"=w861, "Panel controls"=w828, "Standby"=w769) -> ("VD"=w826:dbl[], "Outparams"=w832:T9, "VISA Resource Name out"=w867:refnum<visa-resource-name>, "IS"=w804:dbl[], "ID"=w805:dbl[], "IG"=w803:dbl[], "error out"=w818:errorcluster, "Probe 4"=w829:dbl[])  [unwired: 7 in]
        n212 = Unbundle By Name(w832) -> ("V2 Step"=w831:dbl, "V2 Start"=w830:dbl, "Number of points"=w792:i32)
        n213 = call "4155C Split array.vi"("Number of VAR2 steps"=w792, "Y2 data in"=w805, "X data in"=w826, "Y1 data in"=w804, "Y3 data in"=w803, "error in (no error)"=w818) -> ("Array of clusters"=w819:cluster{"Y data in":dbl[], "X data in":dbl[]}[], "error out"=w780:errorcluster)  [unwired: 1 in]
        n214 = case shown="True" "Plot output curve extrema vs time" {
          tunnel: w825 -> [w888 w958]
          tunnel: w816 -> [w889 w953]
          tunnel: w807 -> [w883 w949]
          tunnel: w806 -> [w882 w948]
          tunnel: w805 -> [_ w945]
          tunnel: w804 -> [_ w943]
          tunnel: w803 -> [_ w942]
          tunnel: w802 -> [w890 w938]
          tunnel: w801 -> [w891 w937]
          tunnel: w800 -> [w886 w934]
          tunnel: w799 -> [w887 w933]
          tunnel: w798 -> [w884 w930]
          tunnel: w797 -> [w885 w929]
          tunnel: w796 -> [w880 w926]
          tunnel: w795 -> [w881 w925]
          tunnel: w794 -> [_ w918]
          tunnel: [w886 w913] -> w793
          tunnel: w792 -> [_ w912]
          tunnel: [w887 w911] -> w791
          tunnel: [w888 w910] -> w790
          tunnel: [w889 w909] -> w789
          tunnel: [w890 w908] -> w788
          tunnel: [w891 w907] -> w787
          tunnel: [w880 w906] -> w786
          tunnel: [w881 w905] -> w785
          tunnel: [w882 w904] -> w784
          tunnel: [w883 w903] -> w783
          tunnel: [w884 w902] -> w782
          tunnel: [w885 w901] -> w781
          tunnel: w780 -> [w892 w900]
          tunnel: [w892 w896] -> w779
          frame False {
          }
          frame True {
            # "Adjusts graph colors."
            # "Adjusts graph colors."
            # "Ion will be the middle element of the array. The calculation of the index is done only once, since Is, Id, and Ig have the same dimensions."
            # "abs(Ig)"
            # "abs(Is)"
            # "Y1: Is\nY2: Id\nY3: Ig"
            # "abs(Id)"
            # "Adjusts graph colors."
            # "Adjusts graph colors."
            # "Adjusts graph colors."
            n215 = Absolute Value(x=w943) -> (abs(x)=w928:dbl[])
            n216 = Absolute Value(x=w945) -> (abs(x)=w944:dbl[])
            n217 = Absolute Value(x=w942) -> (abs(x)=w931:dbl[])
            n218 = Array Size(array=w944) -> (size(s)=w952:i32)
            n219 = Divide(x=w952, y=2) -> (x/y=w895:dbl)
            n220 = Subtract(x=w895, y=1) -> (x-y=w894:dbl)
            n221 = Array Max & Min(array=w928) -> (max value=w935:dbl, min value=w936:dbl)  [unwired: 2 out]
            n222 = Array Max & Min(array=w944) -> (max value=w957:dbl, min value=w941:dbl)  [unwired: 2 out]
            n223 = Array Max & Min(array=w931) -> (max value=w940:dbl, min value=w939:dbl)  [unwired: 2 out]
            n224 = Index Array(array=w928, index=w894) -> (element=w919:dbl)
            n225 = Index Array(array=w928, index=0) -> (element=w920:dbl)
            n226 = Index Array(array=w944, index=w894) -> (element=w921:dbl)
            n227 = Index Array(array=w944, index=0) -> (element=w922:dbl)
            n228 = Index Array(array=w931, index=w894) -> (element=w924:dbl)
            n229 = Index Array(array=w931, index=0) -> (element=w923:dbl)
            n230 = local write "Ig max"(w940) -> ()
            n231 = local write "Ig min"(w939) -> ()
            n232 = local write "Is max"(w935) -> ()
            n233 = local write "Is min"(w936) -> ()
            n234 = local write "Id max"(w957) -> ()
            n235 = local write "Id min"(w941) -> ()
            n236 = Build Array (concatenate)(w934, w935) -> (w913:dbl[])
            n237 = Build Array (concatenate)(w933, w936) -> (w911:dbl[])
            n238 = local write "Is off"(w920) -> ()
            n239 = local write "Is on"(w919) -> ()
            n240 = Build Array (concatenate)(w958, w957) -> (w910:dbl[])
            n241 = Build Array (concatenate)(w953, w941) -> (w909:dbl[])
            n242 = Build Array (concatenate)(w938, w940) -> (w908:dbl[])
            n243 = Build Array (concatenate)(w937, w939) -> (w907:dbl[])
            n244 = Build Array (concatenate)(w926, w919) -> (w906:dbl[])
            n245 = Build Array (concatenate)(w925, w920) -> (w905:dbl[])
            n246 = Build Array (concatenate)(w948, w921) -> (w904:dbl[])
            n247 = Build Array (concatenate)(w949, w922) -> (w903:dbl[])
            n248 = Build Array (concatenate)(w930, w924) -> (w902:dbl[])
            n249 = Build Array (concatenate)(w929, w923) -> (w901:dbl[])
            n250 = local write "Ig off"(w923) -> ()
            n251 = local write "Ig on"(w924) -> ()
            n252 = local write "Id off"(w922) -> ()
            n253 = local write "Id on"(w921) -> ()
            n254 = control-ref of="Imax vs time"() -> (w947:refnum<vi>)
            n255 = control-ref of="Imin vs time"() -> (w946:refnum<vi>)
            n256 = control-ref of="Ion vs time"() -> (w915:refnum<vi>)
            n257 = control-ref of="Ioff vs time"() -> (w914:refnum<vi>)
            n258 = control-ref of="I vs Vg"() -> (w956:refnum<vi>)
            n259 = call "4155C Split array.vi"("Number of VAR2 steps"=w912, "Y2 data in"=w904, "X data in"=w918, "Y1 data in"=w906, "Y3 data in"=w902, "error in (no error)"=w900) -> ("Array of clusters"=w916:cluster{"Y data in":dbl[], "X data in":dbl[]}[], "error out"=w899:errorcluster)  [unwired: 1 in]
            n260 = call "4155C Split array.vi"("Number of VAR2 steps"=w912, "Y2 data in"=w903, "X data in"=w918, "Y1 data in"=w905, "Y3 data in"=w901, "error in (no error)"=w899) -> ("Array of clusters"=w917:cluster{"Y data in":dbl[], "X data in":dbl[]}[], "error out"=w898:errorcluster)  [unwired: 1 in]
            n261 = call "4155C Split array.vi"("Number of VAR2 steps"=w912, "Y2 data in"=w910, "X data in"=w918, "Y1 data in"=w913, "Y3 data in"=w908, "error in (no error)"=w898) -> ("Array of clusters"=w955:cluster{"Y data in":dbl[], "X data in":dbl[]}[], "error out"=w897:errorcluster)  [unwired: 1 in]
            n262 = call "4155C Split array.vi"("Number of VAR2 steps"=w912, "Y2 data in"=w909, "X data in"=w918, "Y1 data in"=w911, "Y3 data in"=w907, "error in (no error)"=w897) -> ("Array of clusters"=w954:cluster{"Y data in":dbl[], "X data in":dbl[]}[], "error out"=w896:errorcluster)  [unwired: 1 in]
            n263 = call "4155C Config Chart Colours.vi"("Numeric"=w912, "XY Graph 2"=w947) -> ()  [unwired: 6 in]
            n264 = call "4155C Config Chart Colours.vi"("Numeric"=w912, "XY Graph 2"=w946) -> ()  [unwired: 6 in]
            n265 = call "4155C Config Chart Colours.vi"("Numeric"=w912, "XY Graph 2"=w915) -> ()  [unwired: 6 in]
            n266 = call "4155C Config Chart Colours.vi"("Numeric"=w912, "XY Graph 2"=w914) -> ()  [unwired: 6 in]
            n267 = call "4155C Config Chart Colours.vi"("Numeric"=w912, "XY Graph 2"=w956) -> ()  [unwired: 6 in]
            n268 = local write "Imax vs time"(w955) -> ()
            n269 = local write "Imin vs time"(w954) -> ()
            n270 = local write "Ion vs time"(w916) -> ()
            n271 = local write "Ioff vs time"(w917) -> ()
          }
        }
        n272 = local write "I vs Vd"(w819) -> ()
        n273 = Open/Create/Replace File(file path (use dialog)=w871, error in=w779, operation (0:open)=w827) -> (refnum out=w814:refnum<file>, error out=w812:errorcluster)  [unwired: 3 in, 1 out]
        n274 = call "4155C Make Big 2d array.vi"("1D Var1"=w826, "1d IS"=w804, "1d ID"=w805, "1d IG"=w803, "1d SMU4"=w829, "SMU4"=w774, "VAR2 START"=w830, "Number of VAR2 steps"=w792, "VAR2 STEP"=w831, "VAR1 Name"="Vd", "Decimal places in header"=i8 1, "VAR2 Name"="Vg") -> ("Header array"=w815:string[], "Data array"=w813:dbl[][])  [unwired: 14 in]
        n275 = call "4155C Write array to file.vi"("Byte Stream File Refnum"=w814, "Header"=w815, "Data Array"=w813, "error in (no error)"=w812) -> ("dup refnum"=w811:refnum<file>, "error out"=w810:errorcluster)  [unwired: 1 in]
        n276 = Close File(refnum=w811, error in=w810) -> (error out=w866:errorcluster)  [unwired: 1 out]
      }
      frame "output-fpp" {
        n277 = local read "FPP - Source"() -> (w963:u32)
        n278 = local read "FPP - Drain"() -> (w964:u32)
        n279 = local read "FPP - Gate"() -> (w965:u32)
        n280 = Number To Decimal String(number=w985) -> (decimal integer string=w1039:string)  [unwired: 1 in]
        n281 = Bundle By Name(cluster=w1015, "Emergency Stop"=w1042) -> (w1052:T1)
        n282 = Delete From Array(array=w1030, index=0 ("Index")) -> (deleted portion=w1028:string, array with subset deleted=w1027:string[])  [unwired: 1 in]
        n283 = VISA Write(VISA resource name=w1006, write buffer=":PAGE:CHAN:MODE SWE;" ("write buffer (\"\")"), error in (no error)=w1003) -> (VISA resource name out=w1005:refnum<visa-resource-name>, error out=w1004:errorcluster)  [unwired: 1 out]
        n284 = Concatenate Strings(w1038, "-outputfpp-" ("Substring"), w1039, w984, ".txt" ("Substring")) -> (w1041:string)
        n285 = case shown="\"d\", Default" w1028 {
          tunnel: [w1053 w1054] -> w1026
          frame "s" {
            w1053 = u16 0 items=["Single", "Double"] ("sweep mode")
          }
          frame "d", Default {
            w1054 = u16 1 items=["Single", "Double"] ("sweep mode")
          }
        }
        n286 = Fract/Exp String To Number(string=w1027) -> (number=w1009:dbl[])  [unwired: 3 in, 1 out]
        n287 = String To Path(string=w1041) -> (path=w1037:path)
        n288 = Index Array(array=w1009, index #1=0 ("Index")) -> (element #1=w1025:dbl, element #2=w1024:dbl, element #3=w1023:dbl)  [unwired: 2 in]
        n289 = Delete From Array(array=w1009, length=3 ("Length"), index=0 ("Index")) -> (array with subset deleted=w1008:dbl[])  [unwired: 1 out]
        n290 = local read "FPP - Probe 1"() -> (w961:u32)
        n291 = local read "FPP - Probe 2"() -> (w962:u32)
        n292 = Bundle By Name(cluster=w1017, "Gate Start"=w1025, "Gate Stop"=w1024, "Gate Step (linear only)"=w1023, "Gate Compliance"=w1035, "Range mode"=w1001, "Range"=w1000) -> (w1051:T6)
        n293 = Index Array(array=w1008, index #1=0 ("Index")) -> (element #1=w1020:dbl, element #2=w1019:dbl, element #3=w1018:dbl)  [unwired: 2 in]
        n294 = call <vilib>:"compatOverwrite.vi"("overwrite (F)"=TRUE) -> ("overwrite?"=w989:T8)
        n295 = Bundle By Name(cluster=w1016, "Drain Start"=w1020, "Drain Stop"=w1019, "Drain Step"=w1018, "Drain Compliance"=w1036, "Range mode"=w999, "Range"=w1002) -> (w1050:T7)
        n296 = call "4155C Output-FPP v2.0.vi"("VISA resource name in"=w1005, "FPP - Source"=w963, "Gate"=w1051, "Drain"=w1050, "FPP - Drain"=w964, "Timings"=w1034, "error in (no error)"=w1004, "FPP - Gate"=w965, "FPP - Probe 1"=w961, "sweep mode"=w1026, "FPP - Probe 2"=w962, "Panel controls"=w1052) -> ("VD"=w994:dbl[], "Outparams"=w997:T9, "VISA Resource Name out"=w1032:refnum<visa-resource-name>, "Vprobe2"=w993:dbl[], "ID"=w992:dbl[], "IG"=w991:dbl[], "Vprobe1"=w990:dbl[], "error out"=w1033:errorcluster)  [unwired: 8 in]
        n297 = Unbundle By Name(w997) -> ("V2 Step"=w998:dbl, "V2 Start"=w996:dbl, "Number of points"=w995:i32)
        n298 = Open/Create/Replace File(file path (use dialog)=w1037, error in=w1033, operation (0:open)=w989) -> (refnum out=w1047:refnum<file>, error out=w1048:errorcluster)  [unwired: 3 in, 1 out]
        n299 = call "4155C Make Big 2d array FPP.vi"("1D Var1"=w994, "1d ID"=w992, "1d Vp2"=w993, "1d IG"=w991, "1d Vp1"=w990, "VAR2 START"=w996, "Number of VAR2 steps"=w995, "VAR2 STEP"=w998, "VAR1 Name"="Vd", "Decimal places in header"=i8 1, "VAR2 Name"="Vg") -> ("Header array"=w1043:string[], "Data array"=w1044:dbl[][])  [unwired: 15 in]
        n300 = call "4155C Write array to file.vi"("Byte Stream File Refnum"=w1047, "Header"=w1043, "Data Array"=w1044, "error in (no error)"=w1048) -> ("dup refnum"=w1045:refnum<file>, "error out"=w1046:errorcluster)  [unwired: 1 in]
        n301 = Close File(refnum=w1045, error in=w1046) -> (error out=w1031:errorcluster)  [unwired: 1 out]
      }
      frame "itime" {
        n302 = Delete From Array(array=w1062, index=1) -> (deleted portion=w1061:string)  [unwired: 1 in, 1 out]
        n303 = Delete From Array(array=w1062, index=0 ("Index")) -> (deleted portion=w1090:string)  [unwired: 1 in, 1 out]
        n304 = Fract/Exp String To Number(string=w1061) -> (number=w1060:dbl)  [unwired: 3 in, 1 out]
        n305 = case shown="\"l\"" w1090 {
          tunnel: w1089 -> [w1095 w1097 w1101]
          tunnel: [w1094 w1096 w1100] -> w1082
          tunnel: w1060 -> [w1092 _ w1099]
          frame "s" {
            w1093 = u32 0 items=["short  ", "medium  ", "long  "] ("integration time 2")
            n306 = Bundle By Name(cluster=w1095, "integration time"=w1093, "Short/Long integration time"=w1092) -> (w1094:T4)
          }
          frame "m", Default {
            w1098 = u32 1 items=["short  ", "medium  ", "long  "] ("integration time 2")
            n307 = Bundle By Name(cluster=w1097, "integration time"=w1098) -> (w1096:T4)
          }
          frame "l" {
            w1102 = u32 2 items=["short  ", "medium  ", "long  "] ("integration time 2")
            n308 = Bundle By Name(cluster=w1101, "integration time"=w1102, "Short/Long integration time"=w1099) -> (w1100:T4)
          }
        }
      }
      frame "pulsed" {
        n309 = Delete From Array(array=w1135, index=0 ("Index")) -> (deleted portion=w1136:string, array with subset deleted=w1123:string[])  [unwired: 1 in]
        n310 = case shown="\"on\", Default" w1136 {
          tunnel: w1134 -> [w1146 w1149]
          tunnel: [w1145 w1148] -> w1127
          tunnel: w1123 -> [w1143 _]
          frame "on", Default {
            w1144 = u16 1 items=["Continuous", "Pulsed"] ("sweep method")
            n311 = Fract/Exp String To Number(string=w1143) -> (number=w1141:dbl[])  [unwired: 3 in, 1 out]
            n312 = Index Array(array=w1141, index #1=0 ("Index")) -> (element #1=w1140:dbl, element #2=w1139:dbl, element #3=w1138:dbl)  [unwired: 2 in]
            n313 = Bundle By Name(cluster=w1146, "sweep method"=w1144, "Pulse period"=w1140, "Base voltage"=w1139, "Pulse width"=w1138) -> (w1145:T4)
          }
          frame "off" {
            w1147 = u16 0 items=["Continuous", "Pulsed"] ("sweep method")
            n314 = Bundle By Name(cluster=w1149, "sweep method"=w1147) -> (w1148:T4)
          }
        }
      }
      frame "gaterangemode" {
        n315 = Delete From Array(array=w1180, index=0 ("Index")) -> (deleted portion=w1181:string)  [unwired: 1 in, 1 out]
        n316 = case shown="\"f\"" w1181 {
          tunnel: [w1183 w1184 w1185] -> w1170
          frame "a", Default {
            w1183 = u16 0 items=["Auto", "Limited", "Fixed"] ("Gate Range\nmode 2")
          }
          frame "f" {
            w1184 = u16 2 items=["Auto", "Limited", "Fixed"] ("Gate Range\nmode 2")
          }
          frame "l" {
            w1185 = u16 1 items=["Auto", "Limited", "Fixed"] ("Gate Range\nmode 2")
          }
        }
      }
      frame "gaterange" {
        (unwired) u8 11 items=["10fA  ", "100fA  ", "1nA  ", "10nA", "100nA", "1uA", "10uA", "100uA", "1mA", "10mA", "100mA", "1A"] ("Gate Range 2")
        n317 = Delete From Array(array=w1223, index=0 ("Index")) -> (deleted portion=w1213:string)  [unwired: 1 in, 1 out]
        n318 = Scan Value(string=w1213, format string="") -> (value=w1211:dbl)  [unwired: 1 in, 1 out]
        n319 = Logarithm Base 10(1:w1211) -> (0:w1210:dbl)
        n320 = Round To Nearest(number=w1210) -> (nearest integer value=w1209:dbl)
        n321 = Add(x=w1209, y=11.0) -> (x+y=w1207:dbl)
        n322 = To Unsigned Byte Integer(number=w1207) -> (unsigned 8bit integer=w1206:u8)
      }
      frame "drainrange" {
        (unwired) u8 11 items=["10fA  ", "100fA  ", "1nA  ", "10nA", "100nA", "1uA", "10uA", "100uA", "1mA", "10mA", "100mA", "1A"] ("Gate Range 2")
        n323 = Delete From Array(array=w1262, index=0 ("Index")) -> (deleted portion=w1253:string)  [unwired: 1 in, 1 out]
        n324 = Scan Value(string=w1253, format string="") -> (value=w1251:dbl)  [unwired: 1 in, 1 out]
        n325 = Logarithm Base 10(1:w1251) -> (0:w1250:dbl)
        n326 = Round To Nearest(number=w1250) -> (nearest integer value=w1249:dbl)
        n327 = Add(x=w1249, y=11.0) -> (x+y=w1247:dbl)
        n328 = To Unsigned Byte Integer(number=w1247) -> (unsigned 8bit integer=w1246:u8)
      }
      frame "drainrangemode" {
        n329 = Delete From Array(array=w1294, index=0 ("Index")) -> (deleted portion=w1295:string)  [unwired: 1 in, 1 out]
        n330 = case shown="\"f\"" w1295 {
          tunnel: [w1297 w1298 w1299] -> w1284
          frame "a", Default {
            w1297 = u16 0 items=["Auto", "Limited", "Fixed"] ("Gate Range\nmode 2")
          }
          frame "f" {
            w1298 = u16 2 items=["Auto", "Limited", "Fixed"] ("Gate Range\nmode 2")
          }
          frame "l" {
            w1299 = u16 1 items=["Auto", "Limited", "Fixed"] ("Gate Range\nmode 2")
          }
        }
      }
      frame "Error", Default {
      }
      frame "logfile" {
        n331 = Number To Decimal String(number=w1350) -> (decimal integer string=w1385:string)  [unwired: 1 in]
        n332 = Concatenate Strings(w1384, "logfile" ("Substring"), w1385, w1348, ".txt" ("Substring")) -> (w1382:string)
        n333 = String To Path(string=w1382) -> (path=w1355:path)
        n334 = Unbundle(w1381) -> ("integration time"=w1380:u32, "Short/Long integration time"=w1379:dbl, "hold time (sec)"=w1378:dbl, "delay time (sec)"=w1377:dbl, "Step Time (0 disables)"=w1376:dbl, "sweep method"=w1375:u16, "Pulse period"=w1374:dbl, "Base voltage"=w1373:dbl, "Pulse width"=w1372:dbl)
        n335 = Build Array(w1380, w1379, w1378, w1377, w1376, w1375, w1374, w1373, w1372, w1366, w1367, w1368, w1369, w1370, w1371) -> (w1359:dbl[])
        n336 = Insert Into Array(array=dbl[][] [] ("Input Array"), new element=w1359) -> (w1358:dbl[][])  [unwired: 2 in]
        n337 = call <vilib>:"compatOverwrite.vi"("overwrite (F)"=TRUE) -> ("overwrite?"=w1353:T8)
        n338 = Open/Create/Replace File(file path (use dialog)=w1355, error in=w1357, operation (0:open)=w1353) -> (refnum out=w1363:refnum<file>, error out=w1362:errorcluster)  [unwired: 3 in, 1 out]
        n339 = call "4155C Write array to file.vi"("Byte Stream File Refnum"=w1363, "Header"=string[] ["Int Time", "Short/Long Itime", "Hold time", "Delay time", "Step time", "Sweep method", "Pulse period", "Base Voltage", "Pulse width", "Drain compliance", "Gate compliance", "Gate range mode", "Gate range", "S/D range mode", "S/D range"], "Data Array"=w1358, "error in (no error)"=w1362) -> ("dup refnum"=w1365:refnum<file>, "error out"=w1364:errorcluster)  [unwired: 1 in]
        n340 = Close File(refnum=w1365, error in=w1364) -> (error out=w1356:errorcluster)  [unwired: 1 out]
      }
      frame "sample" {
        w1407 = 1
        # "Add a time offset (elapsed time) to the time axis."
        # "Adjusts graph colors."
        n341 = Number To Decimal String(number=w1439) -> (decimal integer string=w1481:string)  [unwired: 1 in]
        n342 = Fract/Exp String To Number(string=w1478) -> (number=w1443:dbl[])  [unwired: 3 in, 1 out]
        n343 = local read "Sample - Probe 4"() -> (w1387:u32)
        n344 = Concatenate Strings(w1459, "-sample-" ("Substring"), w1481, w1437, ".txt" ("Substring")) -> (w1479:string)
        n345 = local read "Sample - Drain"() -> (w1388:u32)
        n346 = Index Array(array=w1443, index=0 ("Index")) -> (element=w1476:dbl)
        n347 = String To Path(string=w1479) -> (path=w1463:path)
        n348 = Index Array(array=w1443, index=2 ("Index")) -> (element=w1472:dbl)
        n349 = Index Array(array=w1443, index=3 ("Index")) -> (element=w1445:dbl)
        n350 = Index Array(array=w1443, index=4 ("Index")) -> (element=w1442:dbl)
        n351 = Index Array(array=w1443, index=1 ("Index")) -> (element=w1473:dbl)
        n352 = local read "Plot sample extrema vs time"() -> (w1410:bool)
        n353 = local read "Sample - Gate"() -> (w1390:u32)
        n354 = local read "Sample - Source/Common"() -> (w1389:u32)
        n355 = call "4155C Config Sampling Measurements v2.0.vi"("VISA session"=w1484, "Num Points"=w1472, "Sample - Drain"=w1388, "Display on/off"=TRUE, "Gate Compliance"=w1460, "Sampling interval"=w1442, "Sample - Source/Common"=w1389, "Sample - Probe 4"=w1387, "Drain Compliance"=w1482, "Standby"=w1391, "error in (no error)"=w1483, "Timings"=w1451, "Sample - Gate"=w1390, "Sample time"=w1445) -> ("dup VISA resource name"=w1486:refnum<visa-resource-name>, "error out"=w1485:errorcluster)
        n356 = call "4155C Take Sample v2.0.vi"("VISA resource name in"=w1486, "Emergency Stop"=w1456, "Sample - Gate"=w1390, "Vg"=w1476, "Sample - Drain"=w1388, "Vd"=w1473, "error in (no error)"=w1485) -> ("Time"=w1406:dbl[], "VISA Resource Name out"=w1453:refnum<visa-resource-name>, "Ig"=w1401:dbl[], "Id"=w1402:dbl[], "Is"=w1403:dbl[], "error out"=w1408:errorcluster)  [unwired: 3 in]
        n357 = Insert Into Array(array=w1399, new element=w1402) -> (w1393:dbl[])  [unwired: 1 in]
        n358 = Add(x=w1406, y=w1405) -> (x+y=w1404:dbl[])
        n359 = Insert Into Array(array=w1398, new element=w1403) -> (w1394:dbl[])  [unwired: 1 in]
        n360 = Insert Into Array(array=w1400, new element=w1401) -> (w1396:dbl[])  [unwired: 1 in]
        n361 = case shown="True" w1410 {
          tunnel: w1411 -> [w1487 w1489]
          tunnel: [w1487 w1490] -> w1409
          tunnel: w1404 -> [_ w1488]
          frame False {
          }
          frame True {
            n362 = Insert Into Array(array=w1489, new element=w1488) -> (w1490:i32[])  [unwired: 1 in]
          }
        }
        n363 = case shown="True" "Plot sample extrema vs time" {
          tunnel: w1403 -> [_ w1518]
          tunnel: w1402 -> [_ w1519]
          tunnel: w1401 -> [_ w1520]
          tunnel: [w1497 w1507] -> w1392
          tunnel: w1408 -> [w1497 w1511]
          tunnel: w1432 -> [w1496 w1523]
          tunnel: w1431 -> [w1495 w1522]
          tunnel: w1430 -> [w1494 w1524]
          tunnel: w1429 -> [w1493 w1521]
          tunnel: w1428 -> [w1492 w1526]
          tunnel: w1427 -> [w1491 w1525]
          tunnel: [w1496 w1509] -> w1426
          tunnel: [w1495 w1502] -> w1425
          tunnel: [w1494 w1503] -> w1424
          tunnel: [w1493 w1527] -> w1423
          tunnel: [w1492 w1510] -> w1422
          tunnel: [w1491 w1504] -> w1421
          tunnel: w1409 -> [_ w1498]
          frame False {
          }
          frame True {
            w1505 = 1
            # "Number of VAR2 steps is 1."
            # "abs(Ig)"
            # "abs(Is)"
            # "abs(Id)"
            # "Adjusts graph colors."
            n364 = Absolute Value(x=w1520) -> (abs(x)=w1499:dbl[])
            n365 = Absolute Value(x=w1519) -> (abs(x)=w1500:dbl[])
            n366 = Absolute Value(x=w1518) -> (abs(x)=w1501:dbl[])
            n367 = Array Max & Min(array=w1501) -> (max value=w1517:dbl, min value=w1514:dbl)  [unwired: 2 out]
            n368 = Array Max & Min(array=w1500) -> (max value=w1516:dbl, min value=w1513:dbl)  [unwired: 2 out]
            n369 = Array Max & Min(array=w1499) -> (max value=w1515:dbl, min value=w1512:dbl)  [unwired: 2 out]
            n370 = local write "Id max"(w1516) -> ()
            n371 = local write "Id min"(w1513) -> ()
            n372 = local write "Ig max"(w1515) -> ()
            n373 = local write "Ig min"(w1512) -> ()
            n374 = Insert Into Array(array=w1526, new element=w1499) -> (w1510:dbl[])  [unwired: 1 in]
            n375 = Insert Into Array(array=w1525, new element=w1499) -> (w1504:dbl[])  [unwired: 1 in]
            n376 = local write "Is max"(w1517) -> ()
            n377 = local write "Is min"(w1514) -> ()
            n378 = Insert Into Array(array=w1524, new element=w1500) -> (w1503:dbl[])  [unwired: 1 in]
            n379 = Insert Into Array(array=w1521, new element=w1500) -> (w1527:dbl[])  [unwired: 1 in]
            n380 = Insert Into Array(array=w1523, new element=w1501) -> (w1509:dbl[])  [unwired: 1 in]
            n381 = Insert Into Array(array=w1522, new element=w1501) -> (w1502:dbl[])  [unwired: 1 in]
            n382 = control-ref of="Imax vs time"() -> (w1528:refnum<vi>)
            n383 = call "4155C Config Chart Colours.vi"("Numeric"=w1505, "XY Graph 2"=w1528) -> ()  [unwired: 6 in]
            n384 = call "4155C Split array.vi"("Number of VAR2 steps"=w1505, "Y2 data in"=w1503, "X data in"=w1498, "Y1 data in"=w1509, "Y3 data in"=w1510, "error in (no error)"=w1511) -> ("Array of clusters"=w1529:cluster{"Y data in":dbl[], "X data in":dbl[]}[], "error out"=w1508:errorcluster)  [unwired: 1 in]
            n385 = call "4155C Split array.vi"("Number of VAR2 steps"=w1505, "Y2 data in"=w1503, "X data in"=w1498, "Y1 data in"=w1502, "Y3 data in"=w1504, "error in (no error)"=w1508) -> ("Array of clusters"=w1506:cluster{"Y data in":dbl[], "X data in":dbl[]}[], "error out"=w1507:errorcluster)  [unwired: 1 in]
            n386 = local write "Imax vs time"(w1529) -> ()
            n387 = local write "Imin vs time"(w1506) -> ()
          }
        }
        n388 = Insert Into Array(array=w1397, new element=w1404) -> (w1395:dbl[])  [unwired: 1 in]
        n389 = control-ref of="I vs time (Bias Stress)"() -> (w1414:refnum<vi>)
        n390 = call "4155C Split array.vi"("Number of VAR2 steps"=w1407, "Y2 data in"=w1393, "X data in"=w1395, "Y1 data in"=w1394, "Y3 data in"=w1396) -> ("Array of clusters"=w1413:cluster{"Y data in":dbl[], "X data in":dbl[]}[])  [unwired: 2 in, 1 out]
        n391 = call "4155C Config Chart Colours.vi"("Numeric"=w1407, "XY Graph 2"=w1414) -> ()  [unwired: 6 in]
        n392 = local write "I vs time (Bias Stress)"(w1413) -> ()
        n393 = Insert Into Array(array=dbl[][] [] ("Input Array"), new element=w1404) -> (w1412:dbl[][])  [unwired: 2 in]
        n394 = Insert Into Array(array=w1412, new element=w1401) -> (w1466:dbl[][])  [unwired: 2 in]
        n395 = VISA Write(VISA resource name=w1453, write buffer=":DISP ON" ("write buffer (\"\")"), error in (no error)=w1392) -> (VISA resource name out=w1452:refnum<visa-resource-name>, error out=w1454:errorcluster)  [unwired: 1 out]
        n396 = Insert Into Array(array=w1466, new element=w1402) -> (w1465:dbl[][])  [unwired: 2 in]
        n397 = Insert Into Array(array=w1465, new element=w1403) -> (w1458:dbl[][])  [unwired: 2 in]
        n398 = Transpose 2D Array(2D array=w1458) -> (transposed array=w1457:dbl[][])
        n399 = call <vilib>:"compatOverwrite.vi"("overwrite (F)"=TRUE) -> ("overwrite?"=w1440:T8)
        n400 = Open/Create/Replace File(file path (use dialog)=w1463, error in=w1454, operation (0:open)=w1440) -> (refnum out=w1469:refnum<file>, error out=w1468:errorcluster)  [unwired: 3 in, 1 out]
        n401 = call "4155C Write array to file.vi"("Byte Stream File Refnum"=w1469, "Header"=string[] ["Time /s", "Ig /A", "Id /A", "Is /A"], "Data Array"=w1457, "error in (no error)"=w1468) -> ("dup refnum"=w1471:refnum<file>, "error out"=w1470:errorcluster)  [unwired: 1 in]
        n402 = Close File(refnum=w1471, error in=w1470) -> (error out=w1461:errorcluster)  [unwired: 1 out]
      }
      frame "samplei" {
        n403 = local read "Sample I - Source/Common"() -> (w1530:u32)
        n404 = Number To Decimal String(number=w1555) -> (decimal integer string=w1606:string)  [unwired: 1 in]
        n405 = local read "Sample I - Probe 4 (Disabled)"() -> (w1533:u32)
        n406 = Concatenate Strings(w1585, "-samplei-" ("Substring"), w1606, w1554, ".txt" ("Substring")) -> (w1604:string)
        n407 = Fract/Exp String To Number(string=w1603) -> (number=w1570:dbl[])  [unwired: 3 in, 1 out]
        n408 = String To Path(string=w1604) -> (path=w1588:path)
        n409 = local read "Sample I - Probe 3 (Disabled)"() -> (w1532:u32)
        n410 = Index Array(array=w1570, index=4 ("Index")) -> (element=w1564:dbl)
        n411 = Index Array(array=w1570, index=3 ("Index")) -> (element=w1565:dbl)
        n412 = Index Array(array=w1570, index=1 ("Index")) -> (element=w1567:dbl)
        n413 = Index Array(array=w1570, index=0 ("Index")) -> (element=w1568:dbl)
        n414 = Index Array(array=w1570, index=2 ("Index")) -> (element=w1566:dbl)
        n415 = local read "Sample I - Drain/Gate"() -> (w1531:u32)
        n416 = call "4155C Config SamplingI Measurements v2.0.vi"("VISA session"=w1609, "Num Points"=w1567, "Sample I - Probe 3 (Disabled)"=w1532, "Display on/off"=TRUE, "Sample I - Source/Common"=w1530, "Sample I - Drain/Gate"=w1531, "Sampling interval"=w1565, "Standby"=w1534, "error in (no error)"=w1608, "Timings"=w1577, "Sample I - Probe 4 (Disabled)"=w1533, "Sample time"=w1566) -> ("dup VISA resource name"=w1611:refnum<visa-resource-name>, "error out"=w1610:errorcluster)  [unwired: 2 in]
        n417 = call "4155C Take SampleI v2.0.vi"("Sample I - Drain/Gate"=w1531, "Emergency Stop"=w1582, "error in (no error)"=w1610, "Idg 2"=w1568, "Vdg compliance 2"=w1564, "VISA resource name in"=w1611) -> ("error out"=w1580:errorcluster, "Idg"=w1613:dbl[], "Vdg"=w1590:dbl[], "VISA Resource Name out"=w1578:refnum<visa-resource-name>, "Is"=w1612:dbl[], "Time"=w1594:dbl[])
        n418 = Insert Into Array(array=dbl[][] [] ("Input Array"), new element=w1594) -> (w1593:dbl[][])  [unwired: 2 in]
        n419 = Insert Into Array(array=w1593, new element=w1590) -> (w1592:dbl[][])  [unwired: 2 in]
        n420 = Insert Into Array(array=w1592, new element=w1613) -> (w1591:dbl[][])  [unwired: 2 in]
        n421 = VISA Write(VISA resource name=w1578, write buffer=":DISP ON" ("write buffer (\"\")"), error in (no error)=w1580) -> (VISA resource name out=w1563:refnum<visa-resource-name>, error out=w1579:errorcluster)  [unwired: 1 out]
        n422 = Insert Into Array(array=w1591, new element=w1612) -> (w1584:dbl[][])  [unwired: 2 in]
        n423 = call <vilib>:"compatOverwrite.vi"("overwrite (F)"=TRUE) -> ("overwrite?"=w1558:T8)
        n424 = Open/Create/Replace File(file path (use dialog)=w1588, error in=w1579, operation (0:open)=w1558) -> (refnum out=w1597:refnum<file>, error out=w1596:errorcluster)  [unwired: 3 in, 1 out]
        n425 = Transpose 2D Array(2D array=w1584) -> (transposed array=w1583:dbl[][])
        n426 = call "4155C Write array to file.vi"("Byte Stream File Refnum"=w1597, "Header"=string[] ["Time /s", "Vdg /V", "Idg /A", "Is /A"], "Data Array"=w1583, "error in (no error)"=w1596) -> ("dup refnum"=w1599:refnum<file>, "error out"=w1598:errorcluster)  [unwired: 1 in]
        n427 = Close File(refnum=w1599, error in=w1598) -> (error out=w1561:errorcluster)  [unwired: 1 out]
        n428 = VISA Write(VISA resource name=w1563, write buffer=";:PAGE:SCON:STAN OFF;:PAGE:CHAN:VSU2:DIS;" ("write buffer (\"\")"), error in (no error)=w1561) -> (VISA resource name out=w1559:refnum<visa-resource-name>, error out=w1560:errorcluster)  [unwired: 1 out]
      }
      frame "#" {
        n429 = VISA Write(VISA resource name=w1638, write buffer=":DISP ON" ("write buffer (\"\")"), error in (no error)=w1637) -> (VISA resource name out=w1636:refnum<visa-resource-name>, error out=w1635:errorcluster)  [unwired: 1 out]
      }
      frame "stressV" {
        n430 = Number To Decimal String(number=w1669) -> (decimal integer string=w1710:string)  [unwired: 1 in]
        n431 = Concatenate Strings(w1694, "-stressV-" ("Substring"), w1710, w1668, ".txt" ("Substring")) -> (w1708:string)
        n432 = Fract/Exp String To Number(string=w1707) -> (number=w1680:dbl[])  [unwired: 3 in, 1 out]
        n433 = local read "Stress V - Drain"() -> (w1647:u32)
        n434 = String To Path(string=w1708) -> (path=w1698:path)
        n435 = Index Array(array=w1680, index=3 ("Index")) -> (element=w1677:dbl)
        n436 = Index Array(array=w1680, index=1 ("Index")) -> (element=w1675:dbl)
        n437 = Index Array(array=w1680, index=0 ("Index")) -> (element=w1674:dbl)
        n438 = Index Array(array=w1680, index=4 ("Index")) -> (element=w1679:dbl)
        n439 = Index Array(array=w1680, index=2 ("Index")) -> (element=w1676:dbl)
        n440 = local read "Stress V - Gate"() -> (w1648:u32)
        n441 = local read "Stress V - Source/Common"() -> (w1649:u32)
        n442 = call "4155C Config V Stress v2.0.vi"("Display on/off"=TRUE, "Stress V - Gate"=w1648, "Stress V - Drain"=w1647, "Stress V - Source/Common"=w1649, "IG compliance"=w1676, "ID compliance"=w1677, "error in (no error)"=w1712, "VG"=w1674, "VD"=w1675, "VISA session"=w1713) -> ("error out"=w1714:errorcluster, "dup VISA resource name"=w1715:refnum<visa-resource-name>)
        n443 = call "4155C Apply Stress.vi"("error in (no error)"=w1714, "Duration"=w1679, "Emergency Stop"=w1693, "VISA resource name in"=w1715) -> ("error out"=w1691:errorcluster, "VISA Resource Name out"=w1689:refnum<visa-resource-name>)
        n444 = VISA Write(VISA resource name=w1689, write buffer=":DISP ON" ("write buffer (\"\")"), error in (no error)=w1691) -> (VISA resource name out=w1688:refnum<visa-resource-name>, error out=w1690:errorcluster)  [unwired: 1 out]
        n445 = call <vilib>:"compatOverwrite.vi"("overwrite (F)"=TRUE) -> ("overwrite?"=w1673:T8)
        n446 = Open/Create/Replace File(file path (use dialog)=w1698, error in=w1690, operation (0:open)=w1673) -> (refnum out=w1701:refnum<file>, error out=w1700:errorcluster)  [unwired: 3 in, 1 out]
        n447 = call "4155C Write array to file.vi"("Byte Stream File Refnum"=w1701, "Header"=string[] ["V stress completed successfully", ""], "error in (no error)"=w1700) -> ("dup refnum"=w1703:refnum<file>, "error out"=w1702:errorcluster)  [unwired: 2 in]
        n448 = Close File(refnum=w1703, error in=w1702) -> (error out=w1696:errorcluster)  [unwired: 1 out]
      }
      frame "stressI" {
        n449 = Number To Decimal String(number=w1737) -> (decimal integer string=w1774:string)  [unwired: 1 in]
        n450 = Concatenate Strings(w1758, "-stressI-" ("Substring"), w1774, w1736, ".txt" ("Substring")) -> (w1772:string)
        n451 = Fract/Exp String To Number(string=w1771) -> (number=w1746:dbl[])  [unwired: 3 in, 1 out]
        n452 = local read "Stress I - Source/Common"() -> (w1716:u32)
        n453 = Index Array(array=w1746, index=1 ("Index")) -> (element=w1742:dbl)
        n454 = Index Array(array=w1746, index=0 ("Index")) -> (element=w1743:dbl)
        n455 = Index Array(array=w1746, index=2 ("Index")) -> (element=w1744:dbl)
        n456 = String To Path(string=w1772) -> (path=w1762:path)
        n457 = local read "Stress I - Drain/Gate"() -> (w1717:u32)
        n458 = call "4155C Config I Stress v2.0.vi"("Stress I - Drain/Gate"=w1717, "Stress I - Source/Common"=w1716, "Display on/off"=TRUE, "error in (no error)"=w1776, "VDG compliance"=w1742, "IDG"=w1743, "VISA session"=w1777) -> ("error out"=w1778:errorcluster, "dup VISA resource name"=w1779:refnum<visa-resource-name>)  [unwired: 1 in]
        n459 = call "4155C Apply Stress.vi"("error in (no error)"=w1778, "Duration"=w1744, "Emergency Stop"=w1757, "VISA resource name in"=w1779) -> ("error out"=w1755:errorcluster, "VISA Resource Name out"=w1753:refnum<visa-resource-name>)
        n460 = VISA Write(VISA resource name=w1753, write buffer=":DISP ON" ("write buffer (\"\")"), error in (no error)=w1755) -> (VISA resource name out=w1752:refnum<visa-resource-name>, error out=w1754:errorcluster)  [unwired: 1 out]
        n461 = call <vilib>:"compatOverwrite.vi"("overwrite (F)"=TRUE) -> ("overwrite?"=w1741:T8)
        n462 = Open/Create/Replace File(file path (use dialog)=w1762, error in=w1754, operation (0:open)=w1741) -> (refnum out=w1765:refnum<file>, error out=w1764:errorcluster)  [unwired: 3 in, 1 out]
        n463 = call "4155C Write array to file.vi"("Byte Stream File Refnum"=w1765, "Header"=string[] ["I stress completed successfully", ""], "error in (no error)"=w1764) -> ("dup refnum"=w1767:refnum<file>, "error out"=w1766:errorcluster)  [unwired: 2 in]
        n464 = Close File(refnum=w1767, error in=w1766) -> (error out=w1760:errorcluster)  [unwired: 1 out]
      }
      frame "vsu2pulse" {
        n465 = Number To Decimal String(number=w1800) -> (decimal integer string=w1835:string)  [unwired: 1 in]
        n466 = Concatenate Strings(w1820, "-vsu2-" ("Substring"), w1835, w1799, ".txt" ("Substring")) -> (w1833:string)
        n467 = Fract/Exp String To Number(string=w1832) -> (number=w1808:dbl[])  [unwired: 3 in, 1 out]
        n468 = String To Path(string=w1833) -> (path=w1824:path)
        n469 = Index Array(array=w1808, index=1 ("Index")) -> (element=w1807:dbl)
        n470 = Index Array(array=w1808, index=0 ("Index")) -> (element=w1805:dbl)
        n471 = local read "VSU2 Stress - Source/Common"() -> (w1780:u32)
        n472 = call "4155C Config VSU2 Stress v2.0.vi"("VISA session"=w1838, "Display on/off"=TRUE, "VSU2"=w1805, "error in (no error)"=w1837, "VSU2 Stress - Source/Common"=w1780) -> ("dup VISA resource name"=w1840:refnum<visa-resource-name>, "error out"=w1839:errorcluster)
        n473 = call "4155C Apply Stress.vi"("error in (no error)"=w1839, "Duration"=w1807, "Emergency Stop"=w1819, "VISA resource name in"=w1840) -> ("error out"=w1817:errorcluster, "VISA Resource Name out"=w1815:refnum<visa-resource-name>)
        n474 = VISA Write(VISA resource name=w1815, write buffer=":DISP ON" ("write buffer (\"\")"), error in (no error)=w1817) -> (VISA resource name out=w1814:refnum<visa-resource-name>, error out=w1816:errorcluster)  [unwired: 1 out]
        n475 = call <vilib>:"compatOverwrite.vi"("overwrite (F)"=TRUE) -> ("overwrite?"=w1804:T8)
        n476 = Open/Create/Replace File(file path (use dialog)=w1824, error in=w1816, operation (0:open)=w1804) -> (refnum out=w1827:refnum<file>, error out=w1826:errorcluster)  [unwired: 3 in, 1 out]
        n477 = call "4155C Write array to file.vi"("Byte Stream File Refnum"=w1827, "Header"=string[] ["VSU2 pulse completed successfully", ""], "error in (no error)"=w1826) -> ("dup refnum"=w1829:refnum<file>, "error out"=w1828:errorcluster)  [unwired: 2 in]
        n478 = Close File(refnum=w1829, error in=w1828) -> (error out=w1822:errorcluster)  [unwired: 1 out]
      }
      frame "sample-fpp" {
        w1876 = string[] ["Time /s", "Id VgVd /A", "Ig VgVd /A", "Vp1 VgVd /V", "Vp2 VgVd /V"] ("Header")
        w1880 = "%d" ("format string")
        n479 = local read "FPP - Drain"() -> (w1842:u32)
        n480 = local read "FPP - Source"() -> (w1841:u32)
        n481 = Fract/Exp String To Number(string=w1925) -> (number=w1913:dbl[])  [unwired: 3 in, 1 out]
        n482 = local read "FPP - Probe 1"() -> (w1845:u32)
        n483 = Number To Decimal String(number=w1866) -> (decimal integer string=w1928:string)  [unwired: 1 in]
        n484 = Concatenate Strings(w1919, "-samplefpp-" ("Substring"), w1928, w1865, ".txt" ("Substring")) -> (w1926:string)
        n485 = local read "FPP - Gate"() -> (w1843:u32)
        n486 = String To Path(string=w1926) -> (path=w1888:path)
        n487 = local read "FPP - Probe 2"() -> (w1844:u32)
        n488 = Index Array(array=w1913, index=0 ("Index")) -> (element=w1875:dbl)
        n489 = Index Array(array=w1913, index=1 ("Index")) -> (element=w1874:dbl)
        n490 = Index Array(array=w1913, index=2 ("Index")) -> (element=w1921:dbl)
        n491 = Index Array(array=w1913, index=3 ("Index")) -> (element=w1911:dbl)
        n492 = call "4155C Config Sampling Measurements FPP v2.0.vi"("VISA session"=w1931, "Gate Compliance"=w1920, "FPP - Source"=w1841, "FPP - Drain"=w1842, "Drain Compliance"=w1929, "error in (no error)"=w1930, "Num Points"=w1921, "Timings"=w1918, "FPP - Gate"=w1843, "FPP - Probe 1"=w1845, "Vg"=w1875, "Vd"=w1874, "Display on/off"=TRUE, "Sample time"=w1911, "FPP - Probe 2"=w1844, "Standby"=w1846) -> ("dup VISA resource name"=w1890:refnum<visa-resource-name>, "error out"=w1889:errorcluster)  [unwired: 2 in]
        n493 = Number To Decimal String(number=w1875) -> (decimal integer string=w1900:string)  [unwired: 1 in]
        n494 = call "4155C Take Sample FPP.vi"("VISA resource name in"=w1890, "error in (no error)"=w1889, "Emergency Stop"=w1891) -> ("Time"=w1895:dbl[], "Vp1"=w1905:dbl[], "VISA Resource Name out"=w1872:refnum<visa-resource-name>, "Ig"=w1893:dbl[], "Id"=w1894:dbl[], "Vp2"=w1903:dbl[], "error out"=w1892:errorcluster)  [unwired: 10 in]
        n495 = Insert Into Array(array=dbl[][] [] ("Input Array"), new element=w1895) -> (w1909:dbl[][])  [unwired: 2 in]
        n496 = Number To Decimal String(number=w1874) -> (decimal integer string=w1898:string)  [unwired: 1 in]
        n497 = Insert Into Array(array=w1909, new element=w1894) -> (w1908:dbl[][])  [unwired: 2 in]
        n498 = Concatenate Strings("(Vg = " ("Substring"), w1900, "V, Vd = " ("Substring"), w1898, "V)" ("Substring")) -> (w1896:string)
        n499 = Insert Into Array(array=w1908, new element=w1893) -> (w1907:dbl[][])  [unwired: 2 in]
        n500 = Insert Into Array(array=w1907, new element=w1905) -> (w1904:dbl[][])  [unwired: 2 in]
        n501 = Insert Into Array(array=w1904, new element=w1903) -> (w1873:dbl[][])  [unwired: 2 in]
        n502 = Transpose 2D Array(2D array=w1873) -> (transposed array=w1902:dbl[][])
        n503 = call <vilib>:"compatOverwrite.vi"("overwrite (F)"=TRUE) -> ("overwrite?"=w1870:T8)
        n504 = Open/Create/Replace File(file path (use dialog)=w1888, error in=w1892, operation (0:open)=w1870) -> (refnum out=w1885:refnum<file>, error out=w1886:errorcluster)  [unwired: 3 in, 1 out]
        n505 = Array To Spreadsheet String(array=w1876, 3:w1880) -> (spreadsheet string=w1882:string)  [unwired: 1 in]
        n506 = Search and Replace String(replace all?=TRUE ("replace all? (F)"), input string=w1882, search string="VgVd", replace string=w1896) -> (result string=w1878:string)  [unwired: 4 in, 3 out]
        n507 = Spreadsheet String To Array(format string=w1880, spreadsheet string=w1878, array type (2D Dbl)=w1876) -> (array=w1877:string[])  [unwired: 1 in]
        n508 = call "4155C Write array to file.vi"("Byte Stream File Refnum"=w1885, "Header"=w1877, "Data Array"=w1902, "error in (no error)"=w1886) -> ("dup refnum"=w1883:refnum<file>, "error out"=w1884:errorcluster)  [unwired: 1 in]
        n509 = Close File(refnum=w1883, error in=w1884) -> (error out=w1871:errorcluster)  [unwired: 1 out]
      }
      frame "resample-fpp" {
        w1964 = string[] ["Time /s", "Id VgVd /A", "Ig VgVd /A", "Vp1 VgVd /V", "Vp2 VgVd /V"] ("Header")
        w1968 = "%d" ("format string")
        n510 = Number To Decimal String(number=w1950) -> (decimal integer string=w2008:string)  [unwired: 1 in]
        n511 = Fract/Exp String To Number(string=w2005) -> (number=w1957:dbl[])  [unwired: 3 in, 1 out]
        n512 = Concatenate Strings(w2001, "-resamplefpp-" ("Substring"), w2008, w1951, ".txt" ("Substring")) -> (w2006:string)
        n513 = String To Path(string=w2006) -> (path=w1976:path)
        n514 = Index Array(array=w1957, index=0 ("Index")) -> (element=w1963:dbl)
        n515 = Index Array(array=w1957, index=1 ("Index")) -> (element=w1962:dbl)
        n516 = Number To Decimal String(number=w1963) -> (decimal integer string=w1986:string)  [unwired: 1 in]
        n517 = call "4155C Take Sample FPP.vi"("VISA resource name in"=w1959, "error in (no error)"=w1958, "Emergency Stop"=w1977) -> ("Time"=w1981:dbl[], "Vp1"=w1991:dbl[], "VISA Resource Name out"=w1961:refnum<visa-resource-name>, "Ig"=w1979:dbl[], "Id"=w1980:dbl[], "Vp2"=w1989:dbl[], "error out"=w1978:errorcluster)  [unwired: 10 in]
        n518 = Insert Into Array(array=dbl[][] [] ("Input Array"), new element=w1981) -> (w1995:dbl[][])  [unwired: 2 in]
        n519 = Number To Decimal String(number=w1962) -> (decimal integer string=w1984:string)  [unwired: 1 in]
        n520 = Insert Into Array(array=w1995, new element=w1980) -> (w1994:dbl[][])  [unwired: 2 in]
        n521 = Concatenate Strings("(Vg = " ("Substring"), w1986, "V, Vd = " ("Substring"), w1984, "V)" ("Substring")) -> (w1982:string)
        n522 = Insert Into Array(array=w1994, new element=w1979) -> (w1993:dbl[][])  [unwired: 2 in]
        n523 = Insert Into Array(array=w1993, new element=w1991) -> (w1990:dbl[][])  [unwired: 2 in]
        n524 = Insert Into Array(array=w1990, new element=w1989) -> (w1956:dbl[][])  [unwired: 2 in]
        n525 = call <vilib>:"compatOverwrite.vi"("overwrite (F)"=TRUE) -> ("overwrite?"=w1955:T8)
        n526 = Open/Create/Replace File(file path (use dialog)=w1976, error in=w1978, operation (0:open)=w1955) -> (refnum out=w1973:refnum<file>, error out=w1974:errorcluster)  [unwired: 3 in, 1 out]
        n527 = Array To Spreadsheet String(array=w1964, 3:w1968) -> (spreadsheet string=w1970:string)  [unwired: 1 in]
        n528 = Transpose 2D Array(2D array=w1956) -> (transposed array=w1988:dbl[][])
        n529 = Search and Replace String(replace all?=TRUE ("replace all? (F)"), input string=w1970, search string="VgVd", replace string=w1982) -> (result string=w1966:string)  [unwired: 4 in, 3 out]
        n530 = Spreadsheet String To Array(format string=w1968, spreadsheet string=w1966, array type (2D Dbl)=w1964) -> (array=w1965:string[])  [unwired: 1 in]
        n531 = call "4155C Write array to file.vi"("Byte Stream File Refnum"=w1973, "Header"=w1965, "Data Array"=w1988, "error in (no error)"=w1974) -> ("dup refnum"=w1971:refnum<file>, "error out"=w1972:errorcluster)  [unwired: 1 in]
        n532 = Close File(refnum=w1971, error in=w1972) -> (error out=w1960:errorcluster)  [unwired: 1 out]
      }
      frame "serial" {
        n533 = local read "Termination char\n(0xA = '\\n' = LF)\n(0xD = '\\r' = CR)"() -> (w2035:u8)
        n534 = local read "Enable Termination\nChar (T)"() -> (w2036:bool)
        n535 = Index Array(array=w2043, index=0 ("Index")) -> (element=w2042:string)
        n536 = local read "parity"() -> (w2026:u16)
        n537 = local read "Delay before read (ms)"() -> (w2037:u32)
        n538 = local read "byte count"() -> (w2034:u32)
        n539 = local read "Timeout (ms)"() -> (w2033:u32)
        n540 = local read "VISA resource name"() -> (w2030:refnum<visa-resource-name>)
        n541 = local read "baud rate"() -> (w2029:u32)
        n542 = local read "Serial End Mode for Reads"() -> (w2028:u16)
        n543 = local read "data bits"() -> (w2027:u16)
        n544 = local read "stop bits"() -> (w2032:u16)
        n545 = local read "flow control"() -> (w2031:u16)
        n546 = call "Serial write and read v0.5.vi"("Delay before read (ms)"=w2037, "Termination char\n(0xA = '\\n' = LF)\n(0xD = '\\r' = CR)"=w2035, "Enable Termination\nChar (T)"=w2036, "parity"=w2026, "stop bits"=w2032, "string to write"=w2042, "flow control"=w2031, "byte count"=w2034, "Serial Settings:Serial End Mode for Reads"=w2028, "Timeout (ms)"=w2033, "error in (no error)"=w2048, "VISA resource name"=w2030, "baud rate"=w2029, "data bits"=w2027) -> ("Serial port output"=w2038:string, "error out"=w2047:errorcluster)
        n547 = Build Array (concatenate)(w2038, w2039) -> (w2040:string[])
      }
    }
    n548 = local read "Time Units"() -> (w97:u16)
    n549 = case shown="0" w97 {
      tunnel: ["Time (Seconds)" ("element") "Time (Minutes)" ("element") "Time (Hours)" ("element")] -> w135
      frame 0 {
      }
      frame 1, Default {
      }
      frame 2 {
      }
    }
    n550 = Build Array(w147, w103, w113, w112, w111, w110, w109, w108, w107, w106, w105, w104, w102) -> (w168:dbl[][])
    n551 = Transpose 2D Array(2D array=w168) -> (transposed array=w167:dbl[][])
    n552 = Concatenate Strings(w69, "-Imax_Imin_Ion_Ioff_vs_time.txt" ("Suffix (Imax,Imin,Ion,Ioff)")) -> (w178:string)
    n553 = Build Array(w135, "Is max (A)" ("VAR2 Name"), "Is min (A)" ("VAR2 Name"), "Id max (A)" ("VAR2 Name"), "Id min (A)" ("VAR2 Name"), "Ig max (A)" ("VAR2 Name"), "Ig min (A)" ("VAR2 Name"), "Is on (A)" ("VAR2 Name"), "Is off (A)" ("VAR2 Name"), "Id on (A)" ("VAR2 Name"), "Id off (A)" ("VAR2 Name"), "Ig on (A)" ("VAR2 Name"), "Ig off (A)" ("VAR2 Name")) -> (w173:string[])
    n554 = Array To Spreadsheet String(array=w167, 3:"%e" ("format string")) -> (spreadsheet string=w171:string)  [unwired: 1 in]
    n555 = Array To Spreadsheet String(array=w173, 3:"" ("format string")) -> (spreadsheet string=w172:string)  [unwired: 1 in]
    n556 = String To Path(string=w178) -> (path=w177:path)
    n557 = Build Array(w172, w171) -> (w170:string[])
    n558 = Write to Text File(file (use dialog)=w177, text=w170, error in=w146) -> (refnum out=w179:refnum<file>, error out=w169:errorcluster)  [unwired: 1 in, 1 out]
    n559 = Close File(refnum=w179, error in=w169) -> (error out=w100:errorcluster)  [unwired: 1 out]
    n560 = Concatenate Strings(w69, "-serial_port_output.txt" ("Suffix (serial port log)")) -> (w149:string)
    n561 = String To Path(string=w149) -> (path=w148:path)
    n562 = Build Array(w135, "Serial port input" ("VAR2 Name"), "Serial port output: ") -> (w139:string[])
    n563 = Array To Spreadsheet String(array=w143, 3:"" ("format string")) -> (spreadsheet string=w136:string)  [unwired: 1 in]
    n564 = Array To Spreadsheet String(array=w139, 3:"" ("format string")) -> (spreadsheet string=w137:string)  [unwired: 1 in]
    n565 = Build Array(w137, w136) -> (w138:string[])
    n566 = Array To Spreadsheet String(array=w142, 3:"" ("format string")) -> (spreadsheet string=w154:string)  [unwired: 1 in]
    n567 = Write to Text File(file (use dialog)=w148, text=w138, error in=w100) -> (refnum out=w150:refnum<file>, error out=w151:errorcluster)  [unwired: 1 in, 1 out]
    n568 = Close File(refnum=w150, error in=w151) -> (error out=w71:errorcluster)  [unwired: 1 out]
    n569 = local write "Serial port data"(w154) -> ()
    n570 = Build Array(w68, w67, w66, w65) -> (w81:dbl[][])
    n571 = Build Array("Time (Seconds)" ("element"), "Is (A)" ("VAR2 Name"), "Id (A)" ("VAR2 Name"), "Ig (A)" ("VAR2 Name")) -> (w77:string[])
    n572 = Transpose 2D Array(2D array=w81) -> (transposed array=w80:dbl[][])
    n573 = Concatenate Strings(w69, "-sample_vs_time.txt" ("Suffix (Imax,Imin,Ion,Ioff)")) -> (w87:string)
    n574 = Array To Spreadsheet String(array=w77, 3:"" ("format string")) -> (spreadsheet string=w76:string)  [unwired: 1 in]
    n575 = Array To Spreadsheet String(array=w80, 3:"%e" ("format string")) -> (spreadsheet string=w84:string)  [unwired: 1 in]
    n576 = String To Path(string=w87) -> (path=w86:path)
    n577 = Build Array(w76, w84) -> (w83:string[])
    n578 = Write to Text File(file (use dialog)=w86, text=w83, error in=w71) -> (refnum out=w88:refnum<file>, error out=w82:errorcluster)  [unwired: 1 in, 1 out]
    n579 = Close File(refnum=w88, error in=w82) -> (error out=w70:errorcluster)  [unwired: 1 out]
  }
  "error out" <- w27
  "Timings Indicator" <- w19
  "Probe 4 Indicator" <- w3
  "Is max" <- w13
  "Id max" <- w13
  "Ig max" <- w13
  "Imax vs time" <- w2
  "I vs Vg" <- w2
  "Imin vs time" <- w2
  "I vs Vd" <- w2
  "Serial port data" <- "" ("Serial port data")
  "Is min" <- w12
  "Id min" <- w12
  "Ig min" <- w12
  "Ion vs time" <- w2
  "Ioff vs time" <- w2
  "Is on" <- w11
  "Id on" <- w11
  "Ig on" <- w11
  "Is off" <- w10
  "Id off" <- w10
  "Ig off" <- w10
  "I vs time (Bias Stress)" <- w2
